vi "OP_Print_TPS_cluster0913.vi"() -> ()   [LabVIEW 2013]
uses:
  <vilib>/addons/database/Connection.llb/DB Tools Open Connec (Path).vi
  <vilib>/addons/database/Connection.llb/Conn Execute.vi
  <vilib>/addons/database/Recordset.llb/Rec Fetch Recordset Data (R).vi
  <vilib>/addons/database/Recordset.llb/Rec Destroy - Connection.vi
  <userlib>/caLab/Private/Get_PV-1D.vi
  <userlib>/caLab/Private/Get_PV.vi
  <vilib>/addons/database/NI_Database_API.lvlib
panel:
  in  "last ? Hrs":dbl=12.0 min=1.0 max=24.0 step=1.0
  out "error out 2":errorcluster
  out "x = y?":bool
  out "NOW time":string="21:22:35"
  out "NOW date":string="2017/09/13"
  in  "Save Button":bool
  out "error out 3":errorcluster
  in  "stop":bool
  out "time kickeron":string="21:11:02"
  out "date kickeron":string="2017/09/13"
  out "Cluster":T1={"SR Fill Pattern"=array[864 elements], "Beam Current(mA"=301.29559, "Beam Lifetime(min)"=467.3623843429031, "Beamsize X(um)"=61.81771808059018, "Beamsize Y(um)"=34.43346871436747, "Tune X(from BPM)"=0.0, "Tune Y(from BPM)"=0.0, "Mode"="Top-Up", "NuX(from BBF) "=0.15280663925802224, "NuY(from BBF)"=0.22496346361412184, "IU22-23gap(R)"=7.0, "IU22-05gap(R)"=7.28, "IU22-05M"=TRUE, "IU22A-09gap(R)"=8.058, "IU22A-09M"=TRUE, "IU22B-09gap(R)"=40.001, "IU22B-09M"=FALSE, "IUT22-21gap(R)"=7.0, "IUT22-21M"=TRUE, "IU22-23M"=TRUE, "IU22A-25gap(R)"=7.0, "IU22A-25M"=TRUE, "IU22B-25gap(R)"=40.0, "IU22B-25M"=FALSE, "EPU48A-41gap(R)"=65.0, "EPU48A-41gM"=FALSE, "EPU48B-41gap(R)"=44.99995, "EPU48B-41gM"=TRUE, "EPU46-45gap(R)"=65.00120000000001, "EPU46-45gM"=FALSE, "EPU48A-41phase(R)"=0.0009500000000000001, "EPU48B-41phase(R)"=0.0, "EPU46-45phase(R)"=0.0, "Grid volt.(V)(S)"=33.0, "Gun mode"="MBM", "Mod.3 HV(kV)(S)"=35.519999999999996, "SR"="SR_DMB_2017_0910_1700LOCO.data", "BR"="Booster_JT_2017_0714_1140.data", "Linac"="Linac_2017_0413_1015.data", "LTB"="LTB_JT_2017_0828_1050.data", "BTS"="BTS_2017_0911_0610.data", "RF2 remote"=TRUE, "RF2 OP mode"=TRUE, "RF2 phase.(S)"=-36.2, "RF Freq.(s)"=499655122.5507494, "RF2 gap volt.(S)"=1400.0, "RF3 remote"=TRUE, "RF3 OP mode"=TRUE, "RF3 phase.(S)"=9.000000000000004, "RF3 gap volt.(S)"=1400.0, "BBF V"=TRUE, "BBF H"=TRUE, "BR ext. kicker1(kV)"=17.666, "BR ext. kicker2(kV)"=17.666, "BR ext. sep.1(V)"=322.14, "BR ext. sep.2(V)"=441.1, "BR inj. sep.(V)"=104.95, "BR inj. kicker(kV)"=12.131749999999993, "SR kicker4(kV)"=8.133, "SR kicker3(kV)"=7.798, "SR kicker2(kV)"=8.259, "SR kicker1(kV)"=8.2, "SR inj. sep.2(V)"=397.2, "SR inj. sep.1(V)"=398.04, "Bucket Start"=100.0, "Bucket Last"=600.0, "Bucket Step"=10.0, "Orbit ILK(P)"=TRUE, "IU22-05 Hutch Enable"=TRUE, "IU22A-09M Hutch Enable"=TRUE, "IUT22-21M Hutch Enable"=TRUE, "IU22-23M Hutch Enable"=TRUE, "IU22A-25M Hutch Enable"=TRUE, "EPU48A-41M Hutch Enable"=FALSE, "EPU46-45M Hutch Enable"=FALSE, "EPU46-45 FE Enable"=TRUE, "EPU48A-41 FE Enable"=TRUE, "IU22A-25 FE Enable"=TRUE, "IU22-23 FE Enable"=TRUE, "IUT22-21 FE Enable"=TRUE, "IU22A-09 FE Enable"=TRUE, "IU22-05 FE Enable"=TRUE, "EPU48A-41pM"=FALSE, "EPU48B-41pM"=TRUE, "EPU46-45pM"=FALSE, "Gun volt.(V)(S)"=23.5, "Width count"=30.0, "2ns step"=0.0, "10ps delay"=150.0, "phase shifter"=130.0021, "Taper"=1.0899999999999999, "05XBPMX 1"=-12.071, "09XBPMX 1"=236.232, "21XBPMX 1"=109.949, "23XBPMX 1"=-54.123000000000005, "25XBPMX 1"=836.426, "41XBPMX 1"=-393.619, "45XBPMX 1"=-542.557, "05XBPMY 1"=49.623, "09XBPMY 1"=-49.685, "21XBPMY 1"=1810.249, "23XBPMY 1"=8.221, "25XBPMY 1"=-161.43800000000002, "41XBPMY 1"=188.45000000000002, "45XBPMY 1"=-785.827, "FOFB H"="On", "FOFB V"="On", "time string"="21:22:35", "date"="2017/09/13", "date (last kicker ON)"="2017/09/13", "time string (last kicker ON)"="21:11:02", "BPMX Graph"={[1, 2, 3, 4, 5, 6, 7, 8, 9, 10, 11, 12, 13, 14, 15, 16, 17, 18, 19, 20, 21, 22, 23, 24, 25, 26, 27, 28, 29, 30, 31, 32, 33, 34, 35, 36, 37, 38, 39, 40, 41, 42, 43, 44, 45, 46, 47, 48, 49, 50, 51, 52, 53, 54, 55, 56, 57, 58, 59, 60, 61, 62, 63, 64, 65, 66, 67, 68, 69, 70, 71, 72, 73, 74, 75, 76, 77, 78, 79, 80, 81, 82, 83, 84, 85, 86, 87, 88, 89, 90, 91, 92, 93, 94, 95, 96, 97, 98, 99, 100, 101, 102, 103, 104, 105, 106, 107, 108, 109, 110, 111, 112, 113, 114, 115, 116, 117, 118, 119, 120, 121, 122, 123, 124, 125, 126, 127, 128, 129, 130, 131, 132, 133, 134, 135, 136, 137, 138, 139, 140, 141, 142, 143, 144, 145, 146, 147, 148, 149, 150, 151, 152, 153, 154, 155, 156, 157, 158, 159, 160, 161, 162, 163, 164, 165, 166, 167, 168, 169, 170, 171, 172, 173, 174], "1rst Value (number)"=[-57.953, -16.830000000000002, -69.81400000000001, 33.217, 55.747, -102.116, 112.23700000000001, -53.109, -8.106, -108.797, 42.098, -26.618000000000002, 23.191, -14.290000000000001, -1.155, -135.518, -122.34, 81.94200000000001, -31.955000000000002, -107.23100000000001, 144.648, -41.501, -20.927, -71.483, 72.117, 174.239, 163.291, 218.172, -123.111, -19.648, 721.419, 453.44, -205.66400000000002, 29.594, 134.439, -81.831, 78.56700000000001, 81.661, 6.593, -174.97, 3.722, 159.74, -88.646, 74.924, 15.269, -34.265, -113.105, -24.846, 66.414, -131.589, 93.44500000000001, 99.491, -12.985, -180.05100000000002, 131.165, 37.079, -154.526, 160.38400000000001, 49.599000000000004, 24.96, -73.793, 85.367, 37.467, -10.198, 89.935, -39.093, 45.050000000000004, -60.443, 91.7, -89.60600000000001, -338.463, -13.786, -319.98900000000003, -247.719, -134.31, 117.925, -10.984, -69.336, 71.378, -119.991, 35.43, -76.868, 56.546, -1.875, -582.236, -130.956, -298.747, -39.141, 76.82900000000001, 82.033, -47.447, 68.075, 11.526, -161.376, 200.095, -3.3000000000000003, -170.391, -174.619, -59.896, 50.463, -167.593, 164.144, 6.708, -52.142, -152.178, 67.056, 8.861, -173.928, 197.31, 48.799, -71.952, -62.230000000000004, -4.128, 137.421, -127.104, 79.596, 56.283, -67.373, -122.31400000000001, 36.139, 42.783, -82.897, 55.373000000000005, 14.632, -53.128, -78.393, 32.919000000000004, -27.649, -194.787, 148.28300000000002, 205.038, -156.17600000000002, -87.652, -24.492, 101.044, -122.638, 98.552, 5.809, 62.325, -64.294, 38.297000000000004, 46.068, 274.628, 436.098, -130.642, -298.747, 133.037, 11.423, -153.334, 114.726, 76.023, -90.009, 92.394, 59.627, -74.368, -118.376, 43.591, 66.153, -129.306, 168.713, 4.539, -35.064, -130.217, 42.444, 59.192, -125.98400000000001, 147.53, 66.584, -28.801000000000002, -176.53, 75.164, 77.199, -57.284, -9.878]}, "BPMY Graph"={[1, 2, 3, 4, 5, 6, 7, 8, 9, 10, 11, 12, 13, 14, 15, 16, 17, 18, 19, 20, 21, 22, 23, 24, 25, 26, 27, 28, 29, 30, 31, 32, 33, 34, 35, 36, 37, 38, 39, 40, 41, 42, 43, 44, 45, 46, 47, 48, 49, 50, 51, 52, 53, 54, 55, 56, 57, 58, 59, 60, 61, 62, 63, 64, 65, 66, 67, 68, 69, 70, 71, 72, 73, 74, 75, 76, 77, 78, 79, 80, 81, 82, 83, 84, 85, 86, 87, 88, 89, 90, 91, 92, 93, 94, 95, 96, 97, 98, 99, 100, 101, 102, 103, 104, 105, 106, 107, 108, 109, 110, 111, 112, 113, 114, 115, 116, 117, 118, 119, 120, 121, 122, 123, 124, 125, 126, 127, 128, 129, 130, 131, 132, 133, 134, 135, 136, 137, 138, 139, 140, 141, 142, 143, 144, 145, 146, 147, 148, 149, 150, 151, 152, 153, 154, 155, 156, 157, 158, 159, 160, 161, 162, 163, 164, 165, 166, 167, 168, 169, 170, 171, 172, 173, 174], "1rst Value (number)"=[-151.316, -17.054000000000002, -19.178, 120.799, -59.688, 21.818, 7.809, -29.198, 24.311, 16.134, -40.005, -27.325, 53.925000000000004, 3.1670000000000003, -9.254, 61.293, -34.105000000000004, 94.741, -29.063, -23.54, 22.793, 14.087, -38.574, 36.56, -99.245, -0.044, 48.661, 33.093, -212.454, -68.398, 390.704, 121.525, -58.935, -19.379, 2.579, -18.495, 19.617, -37.129, 48.386, 12.363, -36.386, 3.988, 67.735, -11.383000000000001, 4.172, -13.203, 10.164, -0.589, -22.969, 30.752, -38.915, 41.105000000000004, -21.456, -4.901, 29.631, -9.992, -32.032000000000004, 12.132, -68.125, 97.674, -58.86, 66.602, -68.949, 58.512, -42.012, 22.742, -15.959, 12.297, 5.471, -82.755, 65.11, 15.540000000000001, -166.881, -18.198, 7.187, -10.503, 30.153000000000002, -70.941, -3.086, 7.163, -7.828, -18.855, 26.188, -7.574, 38.271, 0.135, -13.549, 40.546, 139.87800000000001, 4.58, -2.962, -6.871, 5.808, 0.435, 13.713000000000001, -7.65, -7.087, -2.88, 14.262, -32.895, 32.566, -5.7620000000000005, -44.698, 76.731, -22.138, 22.336000000000002, -6.075, -10.424, 12.001, -9.495000000000001, 18.714, -1.697, 7.412, -43.832, 47.095, -41.426, 2.965, 43.068, 29.560000000000002, -31.904, 28.699, -0.466, -7.138, -5.288, -15.559000000000001, 34.502, -45.603, -18.644000000000002, -3.043, -37.238, -6.869, -15.336, -4.0600000000000005, 13.134, -43.802, 53.087, -14.268, -32.236000000000004, 35.516, -16.788, 25.02, -56.714, 59.035000000000004, 117.801, 64.776, -29.192, -39.944, 137.099, -65.81700000000001, 24.237000000000002, -41.801, 16.21, 15.972, -22.743000000000002, 31.377, 18.596, 7.515000000000001, -19.796, 10.161, 1.0070000000000001, -7.114, -12.046, -4.223, 21.048000000000002, -8.239, -20.592, -8.097, 90.321, -136.733, 37.556, 84.604, -63.991, 30.307000000000002, 1.127]}, "Radio Buttons 2"=enum."absolute", "09XBPMX 2"="-47.22", "09XBPMY 2"="-3.76", "05XBPMY 2"="-491.14", "05XBPMX 2"="-472.70", "21XBPMY 2"=" closed", "21XBPMX 2"=" PAB ", "23XBPMY 2"="188.03", "23XBPMX 2"="-8.61", "25XBPMY 2"="5165.53", "25XBPMX 2"="2146.38", "41XBPMY 2"=" closed", "41XBPMX 2"=" Hutch ", "45XBPMX 2"=" Hutch ", "45XBPMY 2"=" closed", "05 mode"="Follow", "09A mode"="Follow", "09B mode"="Follow", "21 mode"="Follow", "23 mode"="Follow", "25A mode"="Follow", "25B mode"="Follow", "41A mode"="Follow", "41B mode"="Follow", "46 mode"="Follow", "BeamCurrent History"={"BPM NO.  1_172"=array[4320 elements], array[4320 elements]}, "SR Beam Current in            hours"=12.0} {"SR Beam Current in            hours" min=1.0 max=24.0 step=1.0 format="%#_2f"; "45XBPMY 1" format="%#.2f"; "41XBPMY 1" format="%#.2f"; "25XBPMY 1" format="%#.2f"; "23XBPMY 1" format="%#.2f"; "21XBPMY 1" format="%#.2f"; "09XBPMY 1" format="%#.2f"; "05XBPMY 1" format="%#.2f"; "45XBPMX 1" format="%#.2f"; "41XBPMX 1" format="%#.2f"; "25XBPMX 1" format="%#.2f"; "23XBPMX 1" format="%#.2f"; "21XBPMX 1" format="%#.2f"; "09XBPMX 1" format="%#.2f"; "05XBPMX 1" format="%#.2f"; "Taper" format="%#.4f"; "phase shifter" format="%#.3f"; "10ps delay" format="%#.1f"; "2ns step" format="%#.1f"; "Width count" format="%#.1f"; "Gun volt.(V)(S)" format="%#.1f"; "Bucket Step" format="%#.2f"; "Bucket Last" format="%#.2f"; "Bucket Start" format="%#.2f"; "BR ext. kicker1(kV)" format="%#.2f"; "BR ext. kicker2(kV)" format="%#.2f"; "BR ext. sep.1(V)" format="%#.2f"; "BR ext. sep.2(V)" format="%#.2f"; "BR inj. sep.(V)" format="%#.3f"; "BR inj. kicker(kV)" format="%#.3f"; "SR kicker4(kV)" format="%#.2f"; "SR kicker3(kV)" format="%#.2f"; "SR kicker2(kV)" format="%#.2f"; "SR kicker1(kV)" format="%#.2f"; "SR inj. sep.2(V)" format="%#.2f"; "SR inj. sep.1(V)" format="%#.2f"; "RF3 gap volt.(S)" format="%#.0f"; "RF3 phase.(S)" format="%#.1f"; "RF2 gap volt.(S)" format="%#.0f"; "RF Freq.(s)" format="%#.1f"; "RF2 phase.(S)" format="%#.1f"; "Mod.3 HV(kV)(S)" format="%#.3f"; "Grid volt.(V)(S)" format="%#.1f"; "EPU46-45phase(R)" format="%#.4f"; "EPU48B-41phase(R)" format="%#.4f"; "EPU48A-41phase(R)" format="%#.4f"; "EPU46-45gap(R)" format="%#.4f"; "EPU48B-41gap(R)" format="%#.4f"; "EPU48A-41gap(R)" format="%#.4f"; "IU22B-25gap(R)" format="%#.4f"; "IU22A-25gap(R)" format="%#.4f"; "IUT22-21gap(R)" format="%#.4f"; "IU22B-09gap(R)" format="%#.4f"; "IU22A-09gap(R)" format="%#.4f"; "IU22-05gap(R)" format="%#.4f"; "IU22-23gap(R)" format="%#.4f"; "NuY(from BBF)" format="%#.4f"; "NuX(from BBF)" format="%#.4f"; "Tune Y(from BPM)" format="%#.4f"; "Tune X(from BPM)" format="%#.4f"; "Beamsize Y(um)" format="%#.2f"; "Beamsize X(um)" format="%#.2f"; "Beam Lifetime(min)" format="%#.3f"; "Beam Current(mA" format="%#.3f"}
  out "date (last Gun ON)":string="2016/08/29"
  out "time string (last Gun ON)":string="23:28:50"
  out "Value Array (number) 7":dbl[](array[numeric])=[-12.071, 49.623, 236.232, -49.685, 109.949, 1810.249, -54.123000000000005, 8.221, 836.426, -161.43800000000002, -393.619, 188.45000000000002, -542.557, -785.827, -472.696, -491.142, -47.215, -3.761, 16.193, -29.476, -8.605, 188.026, 2146.382, 5165.525000000001, -28.331, 10.717, 132.828, -84.862]
  out "Value Array (number) 6":dbl[](array[numeric])=[7.28, 8.058, 40.001, 7.0, 7.0, 7.0, 40.0, 65.0, 0.0009500000000000001, 44.99995, 0.0, 65.00120000000001, 0.0, -1.0899999999999999, 130.0021]
  out "1rst Value (string) 2":string[](array[string])=["MBM", "33", "23.5", "350", "35.52", "22485", "22485", "62", "30", "0", "0", "200", "150"]
  out "Value Array (number) 5":dbl[](array[numeric])=[499654641.19275105, 1.0, 0.0, 1335.005102558433, 1400.0, -56.1, 1.0, 0.0, 1362.1066276040413, 1400.0, 160.0]
  out "1rst Value (string)":string[](array[string])=["Linac_2017_0413_1015.data", "LTB_JT_2017_0828_1050.data", "Booster_JT_2017_0714_1140.data", "BTS_2017_0911_0610.data", "SR_DMB_2017_0910_1700LOCO.data"]
  out "Value Array (number) 4":dbl[](array[numeric])=[499655122.5507494, 1.0, 0.0, 1326.2153542928932, 1400.0, -36.2, 1.0, 0.0, 1398.366426317367, 1400.0, 9.000000000000004]
  out "Value Array (number) 3":dbl[](array[numeric])=[0.0, 33.0, 23.5, 350.0, 35.519999999999996, 22485.0, 22485.0, 62.0, 30.0, 0.0, 0.0, 200.0, 150.0]
  out "Value Array (number) 2":dbl[](array[numeric])=[104.95, 12.131749999999993, 17.666, 17.666, 322.14, 441.1, 398.04, 397.2, 8.2, 8.259, 7.798, 8.133]
  out "Value Array (number)":dbl[](array[numeric])=[1.0, 301.29559, 467.3623843429031, 51.42904998385207, 28.64681257434898, 0.1761252446183953, 0.12524461839530332, 88.36853790283203, 130.0970458984375, 100.0, 600.0, 10.0]
  out "Orbit ILK(A)":bool
  out "Orbit INT. Ang Active":bool
  out "Orbit INT.Ang. On":bool
  out "Orbit INT. Pos Active":bool
  out "Orbit INT.Pos. On":bool
  out "SBM volt.(S)":dbl=350.0 format="%#.1f"
  out "MBM volt.(S)":dbl=23.5 format="%#.1f"
  in  "Copy Button":bool
  in  "Print Button":bool
  in  "Help Button":bool
  in  "Refresh Button":bool
  in  "Open Button":bool
  out "Gun WCM":dbl[](graph)
  out "BR Fill Pattern":dbl[](graph)
  # "TPS OP Handover Information"
  # "Others"
  # "Time："
  # "Valve  Status"
  # "follow"
  # "SM Status"
  # "歷史電流圖\ntrip次數?\n輻射劑量?\n平均氣壓\n目前最高累計劑量\n最近一次觸發時BR電流及WCM數值"
  # "TPS Operational Handover Information v1.3"
  # "SR Status"
  # "Feedback"
  # "Pulse Mag"
  # "LINAC"
  # "x8(ns)"
  # "x2(ns)"
  # "x0.01(ns)"
  # "RF Status"
  # "Hz"
  # "(kV)"
  # "(kV)"
  # "Changeliang@LOP.NSRRC"
  # "SR Fill Pattern"
  # "Lattice Files in using"
  # "ID &Beamline (R)"
  # "mode"
  # "Gap\nmm"
  # "Motor"
  # "Phase"
  # "FE/Hutch"
  # "phase\nshifter"
  # "Taper\n(enc)"
  # "XBPM1X\num"
  # "XBPM1Y\num"
  # "XBPM2X\num"
  # "XBPM2Y\num"
  # "05"
  # "09"
  # "21"
  # "23"
  # "25"
  # "41"
  # "45"
  # "SR Orbit"
  # "BPMX"
  # "BPMY"
  # "SR Beam Current History"
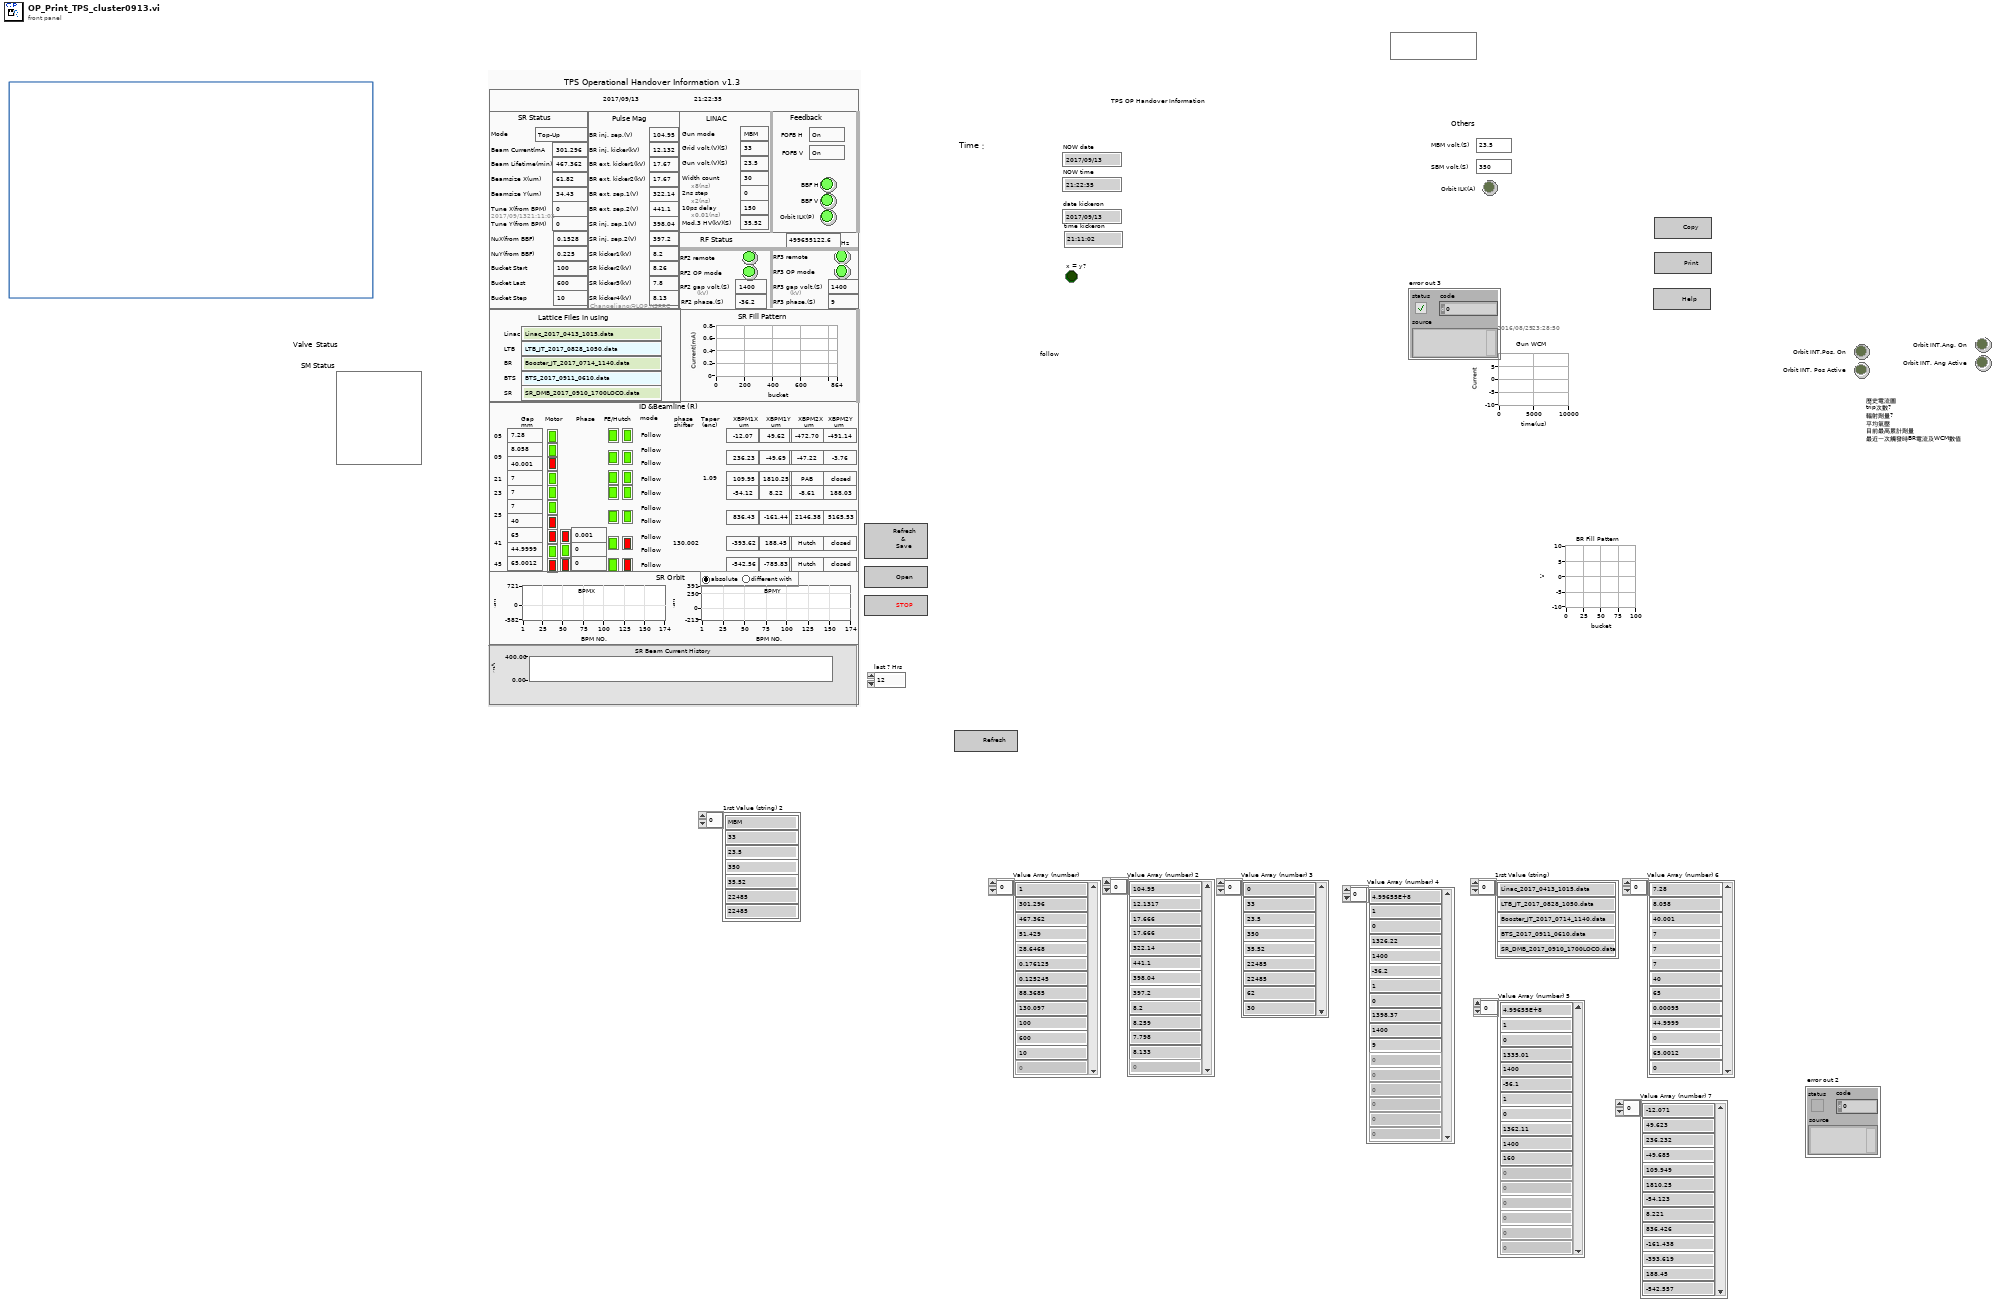
[diagram p1: front panel]
types:
  T1 = cluster{"SR Fill Pattern":dbl[], "Beam Current(mA":dbl, "Beam Lifetime(min)":dbl, "Beamsize X(um)":dbl, "Beamsize Y(um)":dbl, "Tune X(from BPM)":dbl, "Tune Y(from BPM)":dbl, "Mode":string, "NuX(from BBF) ":dbl, "NuY(from BBF)":dbl, "IU22-23gap(R)":dbl, "IU22-05gap(R)":dbl, "IU22-05M":bool, "IU22A-09gap(R)":dbl, "IU22A-09M":bool, "IU22B-09gap(R)":dbl, "IU22B-09M":bool, "IUT22-21gap(R)":dbl, "IUT22-21M":bool, "IU22-23M":bool, "IU22A-25gap(R)":dbl, "IU22A-25M":bool, "IU22B-25gap(R)":dbl, "IU22B-25M":bool, "EPU48A-41gap(R)":dbl, "EPU48A-41gM":bool, "EPU48B-41gap(R)":dbl, "EPU48B-41gM":bool, "EPU46-45gap(R)":dbl, "EPU46-45gM":bool, "EPU48A-41phase(R)":dbl, "EPU48B-41phase(R)":dbl, "EPU46-45phase(R)":dbl, "Grid volt.(V)(S)":dbl, "Gun mode":string, "Mod.3 HV(kV)(S)":dbl, "SR":string, "BR":string, "Linac":string, "LTB":string, "BTS":string, "RF2 remote":bool, "RF2 OP mode":bool, "RF2 phase.(S)":dbl, "RF Freq.(s)":dbl, "RF2 gap volt.(S)":dbl, "RF3 remote":bool, "RF3 OP mode":bool, "RF3 phase.(S)":dbl, "RF3 gap volt.(S)":dbl, "BBF V":bool, "BBF H":bool, "BR ext. kicker1(kV)":dbl, "BR ext. kicker2(kV)":dbl, "BR ext. sep.1(V)":dbl, "BR ext. sep.2(V)":dbl, "BR inj. sep.(V)":dbl, "BR inj. kicker(kV)":dbl, "SR kicker4(kV)":dbl, "SR kicker3(kV)":dbl, "SR kicker2(kV)":dbl, "SR kicker1(kV)":dbl, "SR inj. sep.2(V)":dbl, "SR inj. sep.1(V)":dbl, "Bucket Start":dbl, "Bucket Last":dbl, "Bucket Step":dbl, "Orbit ILK(P)":bool, "IU22-05 Hutch Enable":bool, "IU22A-09M Hutch Enable":bool, "IUT22-21M Hutch Enable":bool, "IU22-23M Hutch Enable":bool, "IU22A-25M Hutch Enable":bool, "EPU48A-41M Hutch Enable":bool, "EPU46-45M Hutch Enable":bool, "EPU46-45 FE Enable":bool, "EPU48A-41 FE Enable":bool, "IU22A-25 FE Enable":bool, "IU22-23 FE Enable":bool, "IUT22-21 FE Enable":bool, "IU22A-09 FE Enable":bool, "IU22-05 FE Enable":bool, "EPU48A-41pM":bool, "EPU48B-41pM":bool, "EPU46-45pM":bool, "Gun volt.(V)(S)":dbl, "Width count":dbl, "2ns step":dbl, "10ps delay":dbl, "phase shifter":dbl, "Taper":dbl, "05XBPMX 1":dbl, "09XBPMX 1":dbl, "21XBPMX 1":dbl, "23XBPMX 1":dbl, "25XBPMX 1":dbl, "41XBPMX 1":dbl, "45XBPMX 1":dbl, "05XBPMY 1":dbl, "09XBPMY 1":dbl, "21XBPMY 1":dbl, "23XBPMY 1":dbl, "25XBPMY 1":dbl, "41XBPMY 1":dbl, "45XBPMY 1":dbl, "FOFB H":string, "FOFB V":string, "time string":string, "date":string, "date (last kicker ON)":string, "time string (last kicker ON)":string, "BPMX Graph":cluster{i32[], "1rst Value (number)":dbl[]}, "BPMY Graph":cluster{i32[], "1rst Value (number)":dbl[]}, "Radio Buttons 2":enum32{"absolute", "different with"}, "09XBPMX 2":string, "09XBPMY 2":string, "05XBPMY 2":string, "05XBPMX 2":string, "21XBPMY 2":string, "21XBPMX 2":string, "23XBPMY 2":string, "23XBPMX 2":string, "25XBPMY 2":string, "25XBPMX 2":string, "41XBPMY 2":string, "41XBPMX 2":string, "45XBPMX 2":string, "45XBPMY 2":string, "05 mode":string, "09A mode":string, "09B mode":string, "21 mode":string, "23 mode":string, "25A mode":string, "25B mode":string, "41A mode":string, "41B mode":string, "46 mode":string, "BeamCurrent History":cluster{"BPM NO.  1_172":dbl[], dbl[]}, "SR Beam Current in            hours":dbl}
  T2 = typedef "NI_Database_API.lvlib/Conn ObjectReference.ctl" = refnum<k1>
  T3 = typedef "NI_Database_API.lvlib/Rec ObjectReference.ctl" = refnum<k1>
  T4 = cluster{"SR Fill Pattern":dbl[], "Beam Current(mA":dbl, "Beam Lifetime(min)":dbl, "Beamsize X(um)":dbl, "Beamsize Y(um)":dbl, "Tune X(from BPM)":dbl, "Tune Y(from BPM)":dbl, "Mode":string, "NuX(from BBF) ":dbl, "NuY(from BBF)":dbl, "IU22-23gap(R)":dbl, "IU22-05gap(R)":dbl, "IU22-05M":bool, "IU22A-09gap(R)":dbl, "IU22A-09M":bool, "IU22B-09gap(R)":dbl, "IU22B-09M":bool, "IUT22-21gap(R)":dbl, "IUT22-21M":bool, "IU22-23M":bool, "IU22A-25gap(R)":dbl, "IU22A-25M":bool, "IU22B-25gap(R)":dbl, "IU22B-25M":bool, "EPU48A-41gap(R)":dbl, "EPU48A-41gM":bool, "EPU48B-41gap(R)":dbl, "EPU48B-41gM":bool, "EPU46-45gap(R)":dbl, "EPU46-45gM":bool, "EPU48A-41phase(R)":dbl, "EPU48B-41phase(R)":dbl, "EPU46-45phase(R)":dbl, "Grid volt.(V)(S)":dbl, "Gun mode":string, "Mod.3 HV(kV)(S)":dbl, "SR":string, "BR":string, "Linac":string, "LTB":string, "BTS":string, "RF2 remote":bool, "RF2 OP mode":bool, "RF2 phase.(S)":dbl, "RF Freq.(s)":dbl, "RF2 gap volt.(S)":dbl, "RF3 remote":bool, "RF3 OP mode":bool, "RF3 phase.(S)":dbl, "RF3 gap volt.(S)":dbl, "BBF V":bool, "BBF H":bool, "BR ext. kicker1(kV)":dbl, "BR ext. kicker2(kV)":dbl, "BR ext. sep.1(V)":dbl, "BR ext. sep.2(V)":dbl, "BR inj. sep.(V)":dbl, "BR inj. kicker(kV)":dbl, "SR kicker4(kV)":dbl, "SR kicker3(kV)":dbl, "SR kicker2(kV)":dbl, "SR kicker1(kV)":dbl, "SR inj. sep.2(V)":dbl, "SR inj. sep.1(V)":dbl, "Bucket Start":dbl, "Bucket Last":dbl, "Bucket Step":dbl, "Orbit ILK(P)":bool, "IU22-05 Hutch Enable":bool, "IU22A-09M Hutch Enable":bool, "IUT22-21M Hutch Enable":bool, "IU22-23M Hutch Enable":bool, "IU22A-25M Hutch Enable":bool, "EPU48A-41M Hutch Enable":bool, "EPU46-45M Hutch Enable":bool, "EPU46-45 FE Enable":bool, "EPU48A-41 FE Enable":bool, "IU22A-25 FE Enable":bool, "IU22-23 FE Enable":bool, "IUT22-21 FE Enable":bool, "IU22A-09 FE Enable":bool, "IU22-05 FE Enable":bool, "EPU48A-41pM":bool, "EPU48B-41pM":bool, "EPU46-45pM":bool, "Gun volt.(V)(S)":dbl, "Width count":dbl, "2ns step":dbl, "10ps delay":dbl, "phase shifter":dbl, "Taper":dbl, "05XBPMX 1":dbl, "09XBPMX 1":dbl, "21XBPMX 1":dbl, "23XBPMX 1":dbl, "25XBPMX 1":dbl, "41XBPMX 1":dbl, "45XBPMX 1":dbl, "05XBPMY 1":dbl, "09XBPMY 1":dbl, "21XBPMY 1":dbl, "23XBPMY 1":dbl, "25XBPMY 1":dbl, "41XBPMY 1":dbl, "45XBPMY 1":dbl, "FOFB H":string, "FOFB V":string, "time string":string, "date":string, "date (last kicker ON)":string, "time string (last kicker ON)":string, "BPMX Graph":cluster{i32[], "1rst Value (number)":dbl[]}, "BPMY Graph":cluster{i32[], "1rst Value (number)":dbl[]}, "Radio Buttons 2":enum32{"absolute", "different with"}, "09XBPMX 2":string, "09XBPMY 2":string, "05XBPMY 2":string, "05XBPMX 2":string, "21XBPMY 2":string, "21XBPMX 2":string, "23XBPMY 2":string, "23XBPMX 2":string, "25XBPMY 2":string, "25XBPMX 2":string, "41XBPMY 2":string, "41XBPMX 2":string, "45XBPMX 2":string, "45XBPMY 2":string, "05 mode":string, "09A mode":string, "09B mode":string, "21 mode":string, "23 mode":string, "25A mode":string, "25B mode":string, "41A mode":string, "41B mode":string, "46 mode":string, "BeamCurrent History":cluster{"BPM NO.  1_172":dbl[], dbl[]}, "SR Beam Current in Last           Hrs":dbl}
  T5 = typedef "imagedata.ctl" = cluster{"image type":i32, "image depth":i32, "image":u8[], "mask":u8[], "colors":u32[], "Rectangle":cluster{"left":i16, "top":i16, "right":i16, "bottom":i16}}
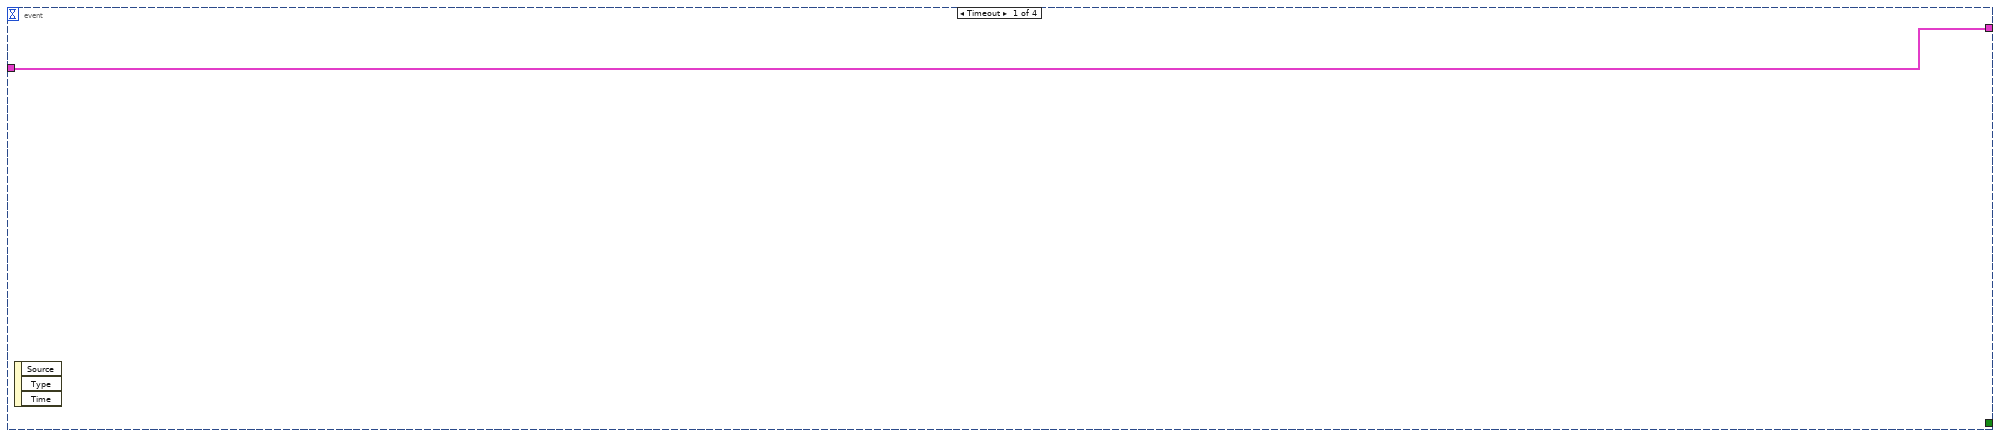
[diagram p4: hidden frame]
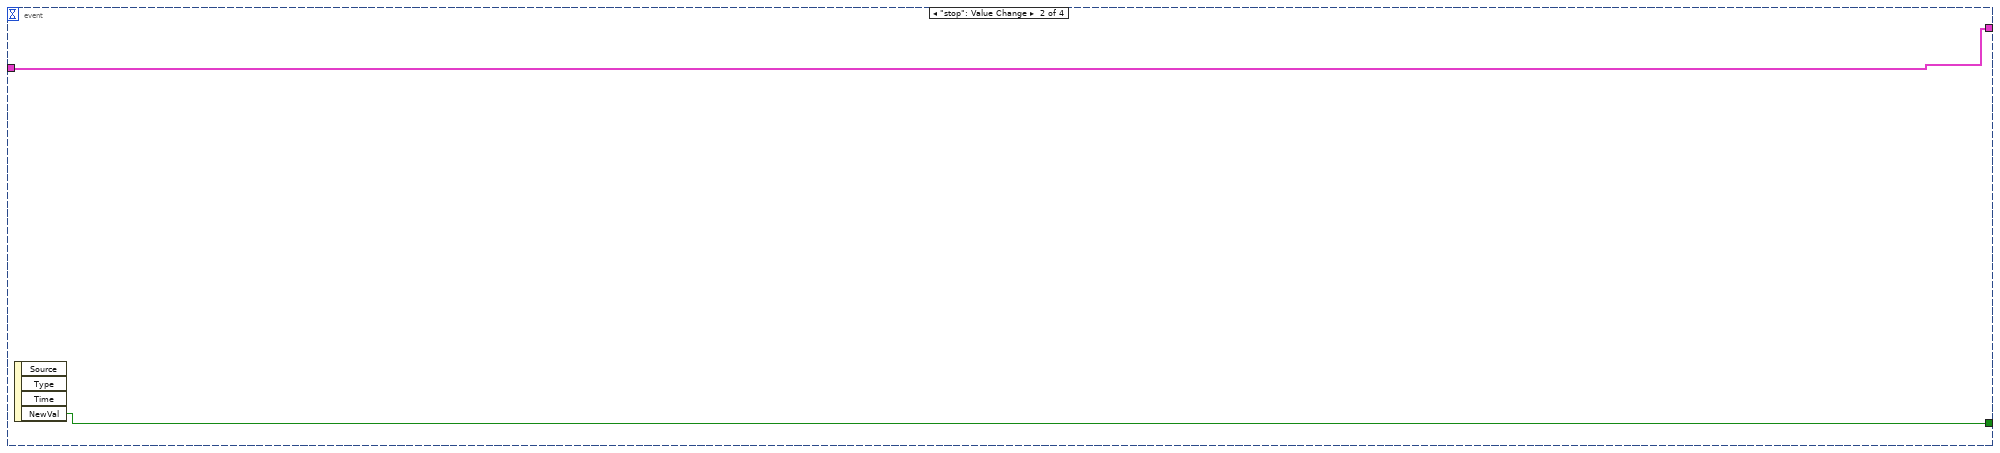
[diagram p5: hidden frame]
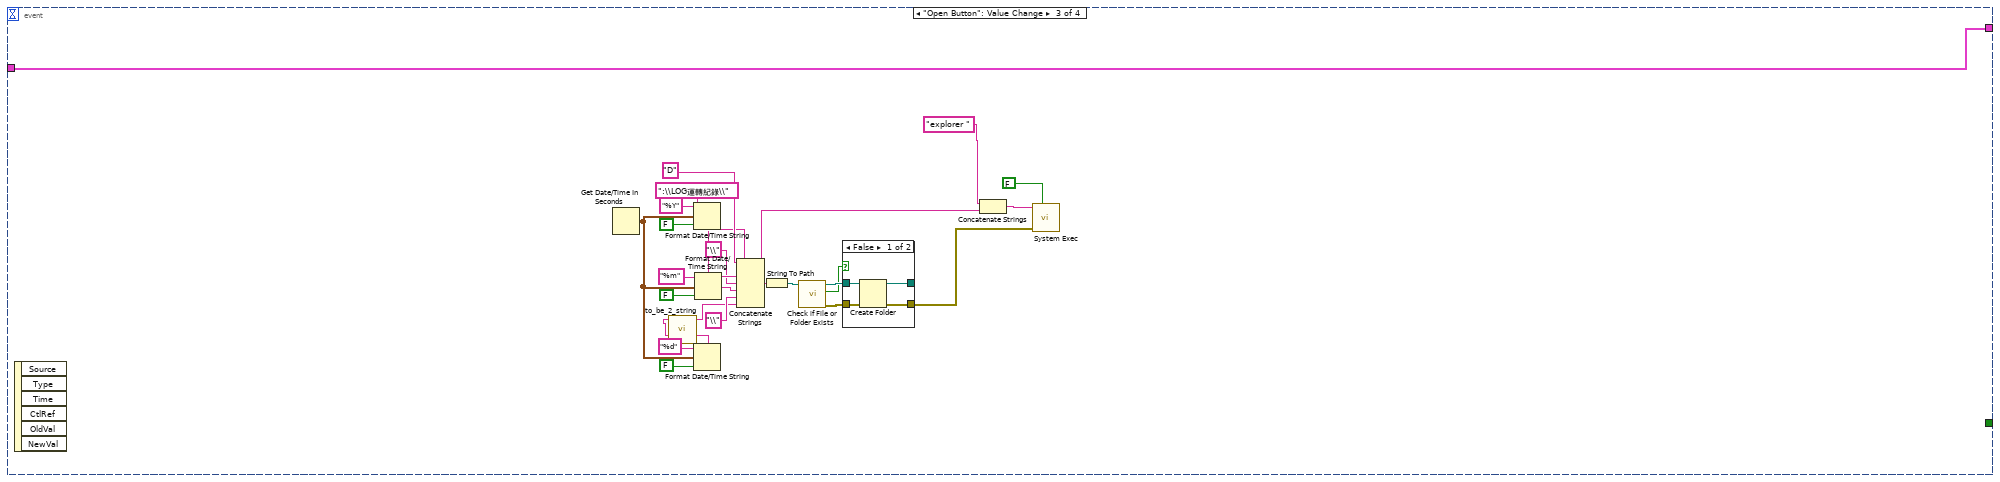
[diagram p6: hidden frame]
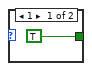
[diagram p9: hidden frame]
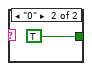
[diagram p12: hidden frame]
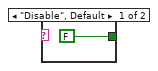
[diagram p13: hidden frame]
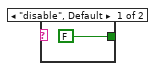
[diagram p14: hidden frame]
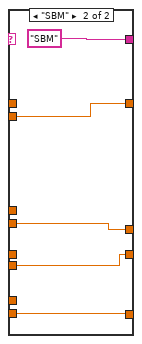
[diagram p15: hidden frame]
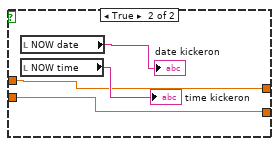
[diagram p16: hidden frame]
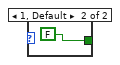
[diagram p17: hidden frame]
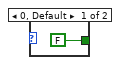
[diagram p18: hidden frame]
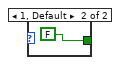
[diagram p19: hidden frame]
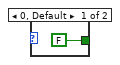
[diagram p20: hidden frame]
diagram:
  (unwired) string[] ["FE-DI-XBPM-051:SA:SA_X_MONITOR", "FE-DI-XBPM-051:SA:SA_Y_MONITOR", "FE-DI-XBPM-091:SA:SA_X_MONITOR", "FE-DI-XBPM-091:SA:SA_Y_MONITOR", "FE-DI-XBPM-211:SA:SA_X_MONITOR", "FE-DI-XBPM-211:SA:SA_Y_MONITOR", "FE-DI-XBPM-231:SA:SA_X_MONITOR", "FE-DI-XBPM-231:SA:SA_Y_MONITOR", "FE-DI-XBPM-251:SA:SA_X_MONITOR", "FE-DI-XBPM-251:SA:SA_Y_MONITOR", "FE-DI-XBPM-411:SA:SA_X_MONITOR", "FE-DI-XBPM-411:SA:SA_Y_MONITOR", "FE-DI-XBPM-451:SA:SA_X_MONITOR", "FE-DI-XBPM-451:SA:SA_Y_MONITOR"]
  (unwired) string[] ["LI-VA-VAL-01:STA:POS", "LI-VA-VAL-02:STA:POS", "LI-VA-VAL-03:STA:POS", "LI-VA-VAL-04:STA:POS", "LI-VA-VAL-05:STA:POS"]
  (unwired) string[] ["SR-DI-SOFB-H:getStatus", "SR-DI-SOFB-V:getStatus", "IGPF:TPSX:FBCTRL", "IGPF:TPSY:FBCTRL", "SR-DI-FOFB-H:getStatus", "SR-DI-FOFB-V:getStatus"]
  # "FE-DI-XBPM-051:SA:SA_Y_MONITOR"
  # "FE-DI-XBPM-051:SA:SA_X_MONITOR"
  # "TPS-SR-052:bpm4:ilk:enabled"
  # "0 為OPEN"
  # "VALVE(EPICS)"
  n1 = local read "last ? Hrs"() -> (w1:dbl)
  n2 = Multiply(x=3600.0 ("y"), y=w1) -> (x*y=w26:dbl)
  n3 = Get Date/Time In Seconds() -> (seconds since 1Jan1904=w36:timestamp)
  n4 = Subtract(x=w36, y=w26) -> (x-y=w35:timestamp)
  n5 = call "TimeToString.vi"("Time Stamp Control"=w36) -> ("result string"=w28:string)
  n6 = call "TimeToString.vi"("Time Stamp Control"=w35) -> ("result string"=w27:string)
  n7 = call <vilib>:"Application Directory.vi"() -> ("Application Directory"=w29:path)
  n8 = Build Path(base path=w29, name or relative path="DSN\\172-18-0-32.dsn") -> (appended path=w31:path)
  n9 = call-poly <vilib>:"DB Tools Open Connection.vi"("connection information"=w31) -> ("error out"=w19:errorcluster, "connection reference"=w18:T2)  [unwired: 7 in]
  n10 = Concatenate Strings("SELECT  float_val , smpl_time\nFROM sample \nwhere  channel_id = 104 and smpl_time between '" ("result string"), w27, "' ::timestamp and '" ("result string"), w28, "' ::timestamp" ("result string")) -> (w3:string)
  n11 = call-poly <vilib>:"DB Tools Execute Query.vi"("error in (no error)"=w19, "SQL query"=w3, "connection reference"=w18) -> ("error out"=w16:errorcluster, "recordset reference"=w17:T3)  [unwired: 5 in]
  n12 = control-ref of="BeamCurrent History"() -> (w32:refnum<vi>)
  n13 = To Double Precision Float(number=w36) -> (double precision float=w33:dbl)
  n14 = To Double Precision Float(number=w35) -> (double precision float=w34:dbl)
  n15 = call-poly <vilib>:"DB Tools Fetch Recordset Data.vi"("error in (no error)"=w16, "recordset reference"=w17) -> ("error out"=w14:errorcluster, "recordset data"=w11:variant[][], "recordset reference out"=w15:T3)  [unwired: 3 in]
  n16 = property on="Property Node" class="XYGraph (strict)"(reference=w32, "XScale.Maximum"=w33, "XScale.Minimum"=w34) -> ()  [unwired: 1 in, 2 out]
  n17 = call-poly <vilib>:"DB Tools Free Object.vi"("error in (no error)"=w14, "recordset reference"=w15) -> ("error out"=w12:errorcluster, "connection reference"=w13:T2)  [unwired: 8 in]
  n18 = Variant To Data(type=string[][] [], Variant=w11) -> (data=w9:string[][])  [unwired: 1 in, 1 out]
  n19 = call <vilib>:"DB Tools Close Connection.vi"("error in (no error)"=w12, "connection reference"=w13) -> ()  [unwired: 5 in, 1 out]
  n20 = Transpose 2D Array(2D array=w9) -> (transposed array=w7:string[][])
  n21 = Index Array(array=w7, index (row) #1=0 ("index (row)"), index (row) #2=1 ("index (row)")) -> (element #1=w21:string[], element #2=w24:string[])  [unwired: 2 in]
  n22 = Fract/Exp String To Number(string=w21) -> (number=w23:dbl[])  [unwired: 3 in, 1 out]
  n23 = for {
    tunnel: w24 -> [w40] mode=indexing
    tunnel: [w39] -> w22 mode=indexing
    n24 = Scan From String "Scan From String"(format string="%<%Y/%m/%d %p %I:%M:%S>T", input string=w40, initial scan location=u32 0, default 1=timestamp(-73814400 s since 1904-01-01)) -> (output 1=w43:timestamp)  [unwired: 1 in, 3 out]
    n25 = To Double Precision Float(number=w43) -> (double precision float=w39:dbl)
  }
  n26 = Bundle(w22, w23) -> (w2:cluster{dbl[], dbl[]})  [unwired: 1 in]
  n27 = while {
    shift-right: [w185] -> _
    shift-left: _ -> [w183]
    shift-right: [w184] -> _
    shift-left: _ -> [w182]
    shift-right: [w45] -> _
    shift-left: w2 -> [w44]
    stop <- "stop" stop-if-true
    w72 = string[] ["SR-ID-IU22-05:setECMode", "SR-ID-IU22A-09:setECMode", "SR-ID-IU22B-09:setECMode", "SR-ID-IUT22-21:setECMode", "SR-ID-IU22-23:setECMode", "SR-ID-IU22A-25:setECMode", "SR-ID-IU22B-25:setECMode", "SR-ID-EPU48A-41:setECMode", "SR-ID-EPU48B-41:setECMode", "SR-ID-EPU46-45:setECMode"]  # ID_mode
    w158 = string[] ["FE-05-PAB:Open", "FE-05-MGV:Open", "FE-05-FCV:Open", "FE-09-PAB:Open", "FE-09-MGV:Open", "FE-09-FCV:Open", "FE-21-PAB:Open", "FE-21-MGV:Open", "FE-21-FCV:Open", "FE-23-PAB:Open", "FE-23-PAB:Open", "FE-23-FCV:Open", "FE-25-PAB:Open", "FE-25-MGV:Open", "FE-25-FCV:Open", "FE-41-PAB:Open", "FE-41-MGV:Open", "FE-41-FCV:Open", "FE-45-PAB:Open", "FE-45-MGV:Open", "FE-45-FCV:Open"]  # PAB_MGV_FCV enable
    (unwired) "LI-DI-WCM:getWfCh1"
    (unwired) "SR-DI-FP:CurrentBuffer"
    w305 = i32[] [1, 2, 3, 4, 5, 6, 7, 8, 9, 10, 11, 12, 13, 14, 15, 16, 17, 18, 19, 20, 21, 22, 23, 24, 25, 26, 27, 28, 29, 30, 31, 32, 33, 34, 35, 36, 37, 38, 39, 40, 41, 42, 43, 44, 45, 46, 47, 48, 49, 50, 51, 52, 53, 54, 55, 56, 57, 58, 59, 60, 61, 62, 63, 64, 65, 66, 67, 68, 69, 70, 71, 72, 73, 74, 75, 76, 77, 78, 79, 80, 81, 82, 83, 84, 85, 86, 87, 88, 89, 90, 91, 92, 93, 94, 95, 96, 97, 98, 99, 100, 101, 102, 103, 104, 105, 106, 107, 108, 109, 110, 111, 112, 113, 114, 115, 116, 117, 118, 119, 120, 121, 122, 123, 124, 125, 126, 127, 128, 129, 130, 131, 132, 133, 134, 135, 136, 137, 138, 139, 140, 141, 142, 143, 144, 145, 146, 147, 148, 149, 150, 151, 152, 153, 154, 155, 156, 157, 158, 159, 160, 161, 162, 163, 164, 165, 166, 167, 168, 169, 170, 171, 172, 173, 174] ("Array 4")
    w303 = 0.001
    w301 = string[] ["SR-DI-BPM-011:Y", "SR-DI-BPM-012:Y", "SR-DI-BPM-013:Y", "SR-DI-BPM-014:Y", "SR-DI-BPM-015:Y", "SR-DI-BPM-016:Y", "SR-DI-BPM-017:Y", "SR-DI-BPM-021:Y", "SR-DI-BPM-022:Y", "SR-DI-BPM-023:Y", "SR-DI-BPM-024:Y", "SR-DI-BPM-025:Y", "SR-DI-BPM-026:Y", "SR-DI-BPM-027:Y", "SR-DI-BPM-031:Y", "SR-DI-BPM-032:Y", "SR-DI-BPM-033:Y", "SR-DI-BPM-034:Y", "SR-DI-BPM-035:Y", "SR-DI-BPM-036:Y", "SR-DI-BPM-037:Y", "SR-DI-BPM-041:Y", "SR-DI-BPM-042:Y", "SR-DI-BPM-043:Y", "SR-DI-BPM-044:Y", "SR-DI-BPM-045:Y", "SR-DI-BPM-046:Y", "SR-DI-BPM-047:Y", "SR-DI-BPM-048:Y", "SR-DI-BPM-050:Y", "SR-DI-BPM-051:Y", "SR-DI-BPM-052:Y", "SR-DI-BPM-053:Y", "SR-DI-BPM-054:Y", "SR-DI-BPM-055:Y", "SR-DI-BPM-056:Y", "SR-DI-BPM-057:Y", "SR-DI-BPM-061:Y", "SR-DI-BPM-062:Y", "SR-DI-BPM-063:Y", "SR-DI-BPM-064:Y", "SR-DI-BPM-065:Y", "SR-DI-BPM-066:Y", "SR-DI-BPM-067:Y", "SR-DI-BPM-071:Y", "SR-DI-BPM-072:Y", "SR-DI-BPM-073:Y", "SR-DI-BPM-074:Y", "SR-DI-BPM-075:Y", "SR-DI-BPM-076:Y", "SR-DI-BPM-077:Y", "SR-DI-BPM-081:Y", "SR-DI-BPM-082:Y", "SR-DI-BPM-083:Y", "SR-DI-BPM-084:Y", "SR-DI-BPM-085:Y", "SR-DI-BPM-086:Y", "SR-DI-BPM-087:Y", "SR-DI-BPM-091:Y", "SR-DI-BPM-092:Y", "SR-DI-BPM-093:Y", "SR-DI-BPM-094:Y", "SR-DI-BPM-095:Y", "SR-DI-BPM-096:Y", "SR-DI-BPM-097:Y", "SR-DI-BPM-101:Y", "SR-DI-BPM-102:Y", "SR-DI-BPM-103:Y", "SR-DI-BPM-104:Y", "SR-DI-BPM-105:Y", "SR-DI-BPM-106:Y", "SR-DI-BPM-107:Y", "SR-DI-BPM-111:Y", "SR-DI-BPM-112:Y", "SR-DI-BPM-113:Y", "SR-DI-BPM-114:Y", "SR-DI-BPM-115:Y", "SR-DI-BPM-116:Y", "SR-DI-BPM-117:Y", "SR-DI-BPM-121:Y", "SR-DI-BPM-122:Y", "SR-DI-BPM-123:Y", "SR-DI-BPM-124:Y", "SR-DI-BPM-125:Y", "SR-DI-BPM-126:Y", "SR-DI-BPM-127:Y", "SR-DI-BPM-128:Y", "SR-DI-BPM-130:Y", "SR-DI-BPM-131:Y", "SR-DI-BPM-132:Y", "SR-DI-BPM-133:Y", "SR-DI-BPM-134:Y", "SR-DI-BPM-135:Y", "SR-DI-BPM-136:Y", "SR-DI-BPM-137:Y", "SR-DI-BPM-141:Y", "SR-DI-BPM-142:Y", "SR-DI-BPM-143:Y", "SR-DI-BPM-144:Y", "SR-DI-BPM-145:Y", "SR-DI-BPM-146:Y", "SR-DI-BPM-147:Y", "SR-DI-BPM-151:Y", "SR-DI-BPM-152:Y", "SR-DI-BPM-153:Y", "SR-DI-BPM-154:Y", "SR-DI-BPM-155:Y", "SR-DI-BPM-156:Y", "SR-DI-BPM-157:Y", "SR-DI-BPM-161:Y", "SR-DI-BPM-162:Y", "SR-DI-BPM-163:Y", "SR-DI-BPM-164:Y", "SR-DI-BPM-165:Y", "SR-DI-BPM-166:Y", "SR-DI-BPM-167:Y", "SR-DI-BPM-171:Y", "SR-DI-BPM-172:Y", "SR-DI-BPM-173:Y", "SR-DI-BPM-174:Y", "SR-DI-BPM-175:Y", "SR-DI-BPM-176:Y", "SR-DI-BPM-177:Y", "SR-DI-BPM-181:Y", "SR-DI-BPM-182:Y", "SR-DI-BPM-183:Y", "SR-DI-BPM-184:Y", "SR-DI-BPM-185:Y", "SR-DI-BPM-186:Y", "SR-DI-BPM-187:Y", "SR-DI-BPM-191:Y", "SR-DI-BPM-192:Y", "SR-DI-BPM-193:Y", "SR-DI-BPM-194:Y", "SR-DI-BPM-195:Y", "SR-DI-BPM-196:Y", "SR-DI-BPM-197:Y", "SR-DI-BPM-201:Y", "SR-DI-BPM-202:Y", "SR-DI-BPM-203:Y", "SR-DI-BPM-204:Y", "SR-DI-BPM-205:Y", "SR-DI-BPM-206:Y", "SR-DI-BPM-207:Y", "SR-DI-BPM-208:Y", "SR-DI-BPM-210:Y", "SR-DI-BPM-211:Y", "SR-DI-BPM-212:Y", "SR-DI-BPM-213:Y", "SR-DI-BPM-214:Y", "SR-DI-BPM-215:Y", "SR-DI-BPM-216:Y", "SR-DI-BPM-217:Y", "SR-DI-BPM-221:Y", "SR-DI-BPM-222:Y", "SR-DI-BPM-223:Y", "SR-DI-BPM-224:Y", "SR-DI-BPM-225:Y", "SR-DI-BPM-226:Y", "SR-DI-BPM-227:Y", "SR-DI-BPM-231:Y", "SR-DI-BPM-232:Y", "SR-DI-BPM-233:Y", "SR-DI-BPM-234:Y", "SR-DI-BPM-235:Y", "SR-DI-BPM-236:Y", "SR-DI-BPM-237:Y", "SR-DI-BPM-241:Y", "SR-DI-BPM-242:Y", "SR-DI-BPM-243:Y", "SR-DI-BPM-244:Y", "SR-DI-BPM-245:Y", "SR-DI-BPM-246:Y", "SR-DI-BPM-247:Y"]  # sorted BPMY_174
    w300 = string[] ["SR-DI-BPM-011:X", "SR-DI-BPM-012:X", "SR-DI-BPM-013:X", "SR-DI-BPM-014:X", "SR-DI-BPM-015:X", "SR-DI-BPM-016:X", "SR-DI-BPM-017:X", "SR-DI-BPM-021:X", "SR-DI-BPM-022:X", "SR-DI-BPM-023:X", "SR-DI-BPM-024:X", "SR-DI-BPM-025:X", "SR-DI-BPM-026:X", "SR-DI-BPM-027:X", "SR-DI-BPM-031:X", "SR-DI-BPM-032:X", "SR-DI-BPM-033:X", "SR-DI-BPM-034:X", "SR-DI-BPM-035:X", "SR-DI-BPM-036:X", "SR-DI-BPM-037:X", "SR-DI-BPM-041:X", "SR-DI-BPM-042:X", "SR-DI-BPM-043:X", "SR-DI-BPM-044:X", "SR-DI-BPM-045:X", "SR-DI-BPM-046:X", "SR-DI-BPM-047:X", "SR-DI-BPM-048:X", "SR-DI-BPM-050:X", "SR-DI-BPM-051:X", "SR-DI-BPM-052:X", "SR-DI-BPM-053:X", "SR-DI-BPM-054:X", "SR-DI-BPM-055:X", "SR-DI-BPM-056:X", "SR-DI-BPM-057:X", "SR-DI-BPM-061:X", "SR-DI-BPM-062:X", "SR-DI-BPM-063:X", "SR-DI-BPM-064:X", "SR-DI-BPM-065:X", "SR-DI-BPM-066:X", "SR-DI-BPM-067:X", "SR-DI-BPM-071:X", "SR-DI-BPM-072:X", "SR-DI-BPM-073:X", "SR-DI-BPM-074:X", "SR-DI-BPM-075:X", "SR-DI-BPM-076:X", "SR-DI-BPM-077:X", "SR-DI-BPM-081:X", "SR-DI-BPM-082:X", "SR-DI-BPM-083:X", "SR-DI-BPM-084:X", "SR-DI-BPM-085:X", "SR-DI-BPM-086:X", "SR-DI-BPM-087:X", "SR-DI-BPM-091:X", "SR-DI-BPM-092:X", "SR-DI-BPM-093:X", "SR-DI-BPM-094:X", "SR-DI-BPM-095:X", "SR-DI-BPM-096:X", "SR-DI-BPM-097:X", "SR-DI-BPM-101:X", "SR-DI-BPM-102:X", "SR-DI-BPM-103:X", "SR-DI-BPM-104:X", "SR-DI-BPM-105:X", "SR-DI-BPM-106:X", "SR-DI-BPM-107:X", "SR-DI-BPM-111:X", "SR-DI-BPM-112:X", "SR-DI-BPM-113:X", "SR-DI-BPM-114:X", "SR-DI-BPM-115:X", "SR-DI-BPM-116:X", "SR-DI-BPM-117:X", "SR-DI-BPM-121:X", "SR-DI-BPM-122:X", "SR-DI-BPM-123:X", "SR-DI-BPM-124:X", "SR-DI-BPM-125:X", "SR-DI-BPM-126:X", "SR-DI-BPM-127:X", "SR-DI-BPM-128:X", "SR-DI-BPM-130:X", "SR-DI-BPM-131:X", "SR-DI-BPM-132:X", "SR-DI-BPM-133:X", "SR-DI-BPM-134:X", "SR-DI-BPM-135:X", "SR-DI-BPM-136:X", "SR-DI-BPM-137:X", "SR-DI-BPM-141:X", "SR-DI-BPM-142:X", "SR-DI-BPM-143:X", "SR-DI-BPM-144:X", "SR-DI-BPM-145:X", "SR-DI-BPM-146:X", "SR-DI-BPM-147:X", "SR-DI-BPM-151:X", "SR-DI-BPM-152:X", "SR-DI-BPM-153:X", "SR-DI-BPM-154:X", "SR-DI-BPM-155:X", "SR-DI-BPM-156:X", "SR-DI-BPM-157:X", "SR-DI-BPM-161:X", "SR-DI-BPM-162:X", "SR-DI-BPM-163:X", "SR-DI-BPM-164:X", "SR-DI-BPM-165:X", "SR-DI-BPM-166:X", "SR-DI-BPM-167:X", "SR-DI-BPM-171:X", "SR-DI-BPM-172:X", "SR-DI-BPM-173:X", "SR-DI-BPM-174:X", "SR-DI-BPM-175:X", "SR-DI-BPM-176:X", "SR-DI-BPM-177:X", "SR-DI-BPM-181:X", "SR-DI-BPM-182:X", "SR-DI-BPM-183:X", "SR-DI-BPM-184:X", "SR-DI-BPM-185:X", "SR-DI-BPM-186:X", "SR-DI-BPM-187:X", "SR-DI-BPM-191:X", "SR-DI-BPM-192:X", "SR-DI-BPM-193:X", "SR-DI-BPM-194:X", "SR-DI-BPM-195:X", "SR-DI-BPM-196:X", "SR-DI-BPM-197:X", "SR-DI-BPM-201:X", "SR-DI-BPM-202:X", "SR-DI-BPM-203:X", "SR-DI-BPM-204:X", "SR-DI-BPM-205:X", "SR-DI-BPM-206:X", "SR-DI-BPM-207:X", "SR-DI-BPM-208:X", "SR-DI-BPM-210:X", "SR-DI-BPM-211:X", "SR-DI-BPM-212:X", "SR-DI-BPM-213:X", "SR-DI-BPM-214:X", "SR-DI-BPM-215:X", "SR-DI-BPM-216:X", "SR-DI-BPM-217:X", "SR-DI-BPM-221:X", "SR-DI-BPM-222:X", "SR-DI-BPM-223:X", "SR-DI-BPM-224:X", "SR-DI-BPM-225:X", "SR-DI-BPM-226:X", "SR-DI-BPM-227:X", "SR-DI-BPM-231:X", "SR-DI-BPM-232:X", "SR-DI-BPM-233:X", "SR-DI-BPM-234:X", "SR-DI-BPM-235:X", "SR-DI-BPM-236:X", "SR-DI-BPM-237:X", "SR-DI-BPM-241:X", "SR-DI-BPM-242:X", "SR-DI-BPM-243:X", "SR-DI-BPM-244:X", "SR-DI-BPM-245:X", "SR-DI-BPM-246:X", "SR-DI-BPM-247:X"]  # sorted BPMX_174
    w360 = string[] ["BL-05A:HutchA_Enable", "BL-09A:HutchA_Enable", "BL-21A:HutchA_Enable", "BL-23A:HutchA_Enable", "BL-25A:HutchA_Enable", "BL-41A:HutchA_Enable", "BL-45A:HutchA_Enable"]  # Hutch enable
    w379 = string[] ["CPCI03-adl7452-0:doBank0Ch5", "CPCI05-adl7452-0:doBank0Ch5", "CPCI11-adl7452-0:doBank0Ch5", "CPCI12-adl7452-0:doBank0Ch5", "CPCI13-adl7452-0:doBank0Ch5", "CPCI21-adl7452-0:doBank0Ch5", "CPCI23-adl7452-0:doBank0Ch5"]  # FE enable
    (unwired) 1 ("index")
    w456 = 578.303 ("y")
    w461 = 1.202 ("y")
    # "D:\\LOG運轉紀錄\\2016"
    # "45"
    # "41"
    # "25"
    # "23"
    # "21"
    # "09"
    # "05"
    # "0為"
    # "05\n09\n21\n23\n25\n41\n45"
    # "gapMotorOff"
    n28 = disable-structure shown="Disabled" {
      frame Disabled {
        n29 = call-poly <userlib>:"CaLabGet.vi"("PV Name"="TI-INJ-PROC:getTrig-LI-EGUN") -> ("1rst Value (string)"=w621:string)  [unwired: 8 in, 6 out]
        n30 = Equal?(x="1" ("1rst Value (string)"), y=w621) -> (x = y?=w619:bool)
        n31 = case shown="True" w619 {
          frame False {
          }
          frame True {
            n32 = local read item#-1() -> (→"date (last Gun ON)")
            n33 = local read item#-1() -> (→"time string (last Gun ON)")
          }
        }
      }
      frame Enabled {
      }
    }
    n34 = event shown="[3] \"Save Button\": Value Change" {
      selector: _ -> [_ _ _ _]
      dyn-events: _ -> [_ _ _ _]
      timeout: 233 -> [_ _ _ _]
      tunnel: [_ w484 _ _] -> w46
      tunnel: [w482 w483 w485 w522] -> w45
      tunnel: w44 -> [w482 w483 w485 _]
      event Timeout {
        n35 = event-data() -> ()  [unwired: 1 in, 3 out]
      }
      event "stop": Value Change {
        n36 = event-data() -> ("NewVal"=w484:bool)  [unwired: 1 in, 3 out]
      }
      event "Open Button": Value Change {
        n37 = event-data() -> ()  [unwired: 1 in, 6 out]
        n38 = Get Date/Time In Seconds() -> (seconds since 1Jan1904=w506:timestamp)
        n39 = Format Date/Time String(time format string (%c)="%Y", seconds (now)=w506, UTC format=FALSE) -> (date/time string=w498:string)
        n40 = Format Date/Time String(time format string (%c)="%d", seconds (now)=w506, UTC format=FALSE) -> (date/time string=w489:string)
        n41 = call "to_be_2_string.vi"("string 2"=w489) -> ("substring 2"=w488:string)  [unwired: 10 in]
        n42 = Format Date/Time String(time format string (%c)="%m", seconds (now)=w506, UTC format=FALSE) -> (date/time string=w494:string)
        n43 = Concatenate Strings("D" ("磁碟位置"), ":\\LOG運轉紀錄\\", w498, "\\", w494, "\\", w488) -> (w486:string)
        n44 = String To Path(string=w486) -> (path=w502:path)
        n45 = call <vilib>:"Check if File or Folder Exists.vi"("path"=w502) -> ("error out"=w504:errorcluster, "file or folder exists?"=w490:bool, "dup path"=w503:path)  [unwired: 8 in]
        n46 = case shown="False" w490 {
          tunnel: w503 -> [w513 w515]
          tunnel: w504 -> [w512 w514]
          tunnel: [w511 w515] -> _
          tunnel: [w510 w514] -> w487
          frame False {
            n47 = Create Folder(path (use dialog)=w513, error in=w512) -> (created path=w511:path, error out=w510:errorcluster)  [unwired: 1 in, 1 out]
          }
          frame True {
          }
        }
        n48 = Concatenate Strings("explorer ", w486) -> (w508:string)
        n49 = call <vilib>:"System Exec.vi"("wait until completion? (T)"=FALSE, "error in (no error)"=w487, "command line"=w508) -> ()  [unwired: 5 in, 4 out]
      }
      event "Save Button": Value Change {
        n50 = event-data() -> ()  [unwired: 1 in, 1 out]
        n51 = flat-sequence {
          tunnel: [w525] -> w520
          tunnel: [w524] -> w519
          tunnel: [w523] -> w518
          tunnel: [w565] -> w521
          tunnel: w520 -> [w565]
          tunnel: w519 -> [w563]
          tunnel: w518 -> [w564]
          tunnel: [w564] -> w517
          tunnel: [w563] -> w516
          tunnel: [w572] -> w522
          tunnel: w521 -> [w572]
          tunnel: w517 -> [w568]
          tunnel: w516 -> [w567]
          frame #0 {
            n52 = Multiply(x=3600.0 ("y"), y="last ? Hrs") -> (x*y=w533:dbl)
            n53 = Get Date/Time In Seconds() -> (seconds since 1Jan1904=w523:timestamp)
            n54 = Subtract(x=w523, y=w533) -> (x-y=w524:timestamp)
            n55 = call "TimeToString.vi"("Time Stamp Control"=w523) -> ("result string"=w531:string)
            n56 = call "TimeToString.vi"("Time Stamp Control"=w524) -> ("result string"=w532:string)
            n57 = call <vilib>:"Application Directory.vi"() -> ("Application Directory"=w530:path)
            n58 = Build Path(base path=w530, name or relative path="DSN\\172-18-0-32.dsn") -> (appended path=w528:path)
            n59 = call-poly <vilib>:"DB Tools Open Connection.vi"("connection information"=w528) -> ("error out"=w540:errorcluster, "connection reference"=w541:T2)  [unwired: 7 in]
            n60 = Concatenate Strings("SELECT  float_val , smpl_time\nFROM sample \nwhere  channel_id = 104 and smpl_time between '" ("result string"), w532, "' ::timestamp and '" ("result string"), w531, "' ::timestamp" ("result string")) -> (w556:string)
            n61 = call-poly <vilib>:"DB Tools Execute Query.vi"("error in (no error)"=w540, "SQL query"=w556, "connection reference"=w541) -> ("error out"=w543:errorcluster, "recordset reference"=w542:T3)  [unwired: 5 in]
            n62 = call-poly <vilib>:"DB Tools Fetch Recordset Data.vi"("error in (no error)"=w543, "recordset reference"=w542) -> ("error out"=w545:errorcluster, "recordset data"=w548:variant[][], "recordset reference out"=w544:T3)  [unwired: 3 in]
            n63 = call-poly <vilib>:"DB Tools Free Object.vi"("error in (no error)"=w545, "recordset reference"=w544) -> ("error out"=w547:errorcluster, "connection reference"=w546:T2)  [unwired: 8 in]
            n64 = Variant To Data(type=string[][] [], Variant=w548) -> (data=w550:string[][])  [unwired: 1 in, 1 out]
            n65 = call <vilib>:"DB Tools Close Connection.vi"("error in (no error)"=w547, "connection reference"=w546) -> ("error out"=→"error out 2":errorcluster)  [unwired: 5 in]
            n66 = Transpose 2D Array(2D array=w550) -> (transposed array=w552:string[][])
            n67 = Index Array(array=w552, index (row) #1=0 ("index (row)"), index (row) #2=1 ("index (row)")) -> (element #1=w538:string[], element #2=w535:string[])  [unwired: 2 in]
            n68 = for {
              tunnel: w535 -> [w559] mode=indexing
              tunnel: [w558] -> w537 mode=indexing
              n69 = Scan From String "Scan From String"(format string="%<%Y/%m/%d %p %I:%M:%S>T", input string=w559, initial scan location=u32 0, default 1=timestamp(-73814400 s since 1904-01-01)) -> (output 1=w562:timestamp)  [unwired: 1 in, 3 out]
              n70 = To Double Precision Float(number=w562) -> (double precision float=w558:dbl)
            }
            n71 = Fract/Exp String To Number(string=w538) -> (number=w536:dbl[])  [unwired: 3 in, 1 out]
            n72 = Bundle(w537, w536) -> (w525:cluster{dbl[], dbl[]})  [unwired: 1 in]
          }
          frame #1 {
            n73 = Wait (ms)(milliseconds to wait=u32 300) -> ()  [unwired: 1 out]
          }
          frame #2 {
            n74 = Get Date/Time In Seconds() -> (seconds since 1Jan1904=w575:timestamp)
            n75 = Format Date/Time String(time format string (%c)="%Y", seconds (now)=w575, UTC format=FALSE) -> (date/time string=w594:string)
            n76 = Format Date/Time String(time format string (%c)="%d", seconds (now)=w575, UTC format=FALSE) -> (date/time string=w603:string)
            n77 = call "to_be_2_string.vi"("string 2"=w603) -> ("substring 2"=w604:string)  [unwired: 10 in]
            n78 = Format Date/Time String(time format string (%c)="%m", seconds (now)=w575, UTC format=FALSE) -> (date/time string=w598:string)
            n79 = Format Date/Time String(time format string (%c)="%Y%m%d%H%M%S", seconds (now)=w575) -> (date/time string=w582:string)  [unwired: 1 in]
            n80 = Concatenate Strings("D" ("磁碟位置"), ":\\LOG運轉紀錄\\", w594, "\\", w598, "\\", w604) -> (w587:string)
            n81 = String To Path(string=w587) -> (path=w590:path)
            n82 = call <vilib>:"Check if File or Folder Exists.vi"("path"=w590) -> ("error out"=w588:errorcluster, "file or folder exists?"=w602:bool, "dup path"=w589:path)  [unwired: 8 in]
            n83 = invoke on="Cluster" class="Clust (strict)" method="Get Image"() -> ("image data"=w573:T5)  [unwired: 6 in, 5 out]
            n84 = case shown="False" w602 {
              tunnel: w589 -> [w608 w610]
              tunnel: w588 -> [w607 w609]
              tunnel: [w606 w610] -> w574
              tunnel: [w605 w609] -> _
              frame False {
                n85 = Create Folder(path (use dialog)=w608, error in=w607) -> (created path=w606:path, error out=w605:errorcluster)  [unwired: 1 in, 1 out]
              }
              frame True {
              }
            }
            n86 = Path To String(path=w574) -> (string=w586:string)
            n87 = control-ref of="BeamCurrent History"() -> (w571:refnum<vi>)
            n88 = To Double Precision Float(number=w568) -> (double precision float=w570:dbl)
            n89 = To Double Precision Float(number=w567) -> (double precision float=w569:dbl)
            n90 = Concatenate Strings(w586, "\\" ("string"), w582) -> (w576:string)
            n91 = property on="Property Node" class="XYGraph (strict)"(reference=w571, "XScale.Maximum"=w570, "XScale.Minimum"=w569) -> ()  [unwired: 1 in, 2 out]
            n92 = Concatenate Strings(w576, ".jpg" ("file format")) -> (w577:string)
            n93 = String To Path(string=w577) -> (path=w581:path)
            n94 = call <vilib>:"Write JPEG File.vi"("quality (80)"=100, "image data"=w573, "path to JPEG file"=w581) -> ("error out"=→"error out 3":errorcluster)  [unwired: 7 in, 1 out]
          }
        }
      }
    }
    n95 = disable-structure shown="Disabled" {
      frame Disabled {
        n96 = Bundle By Name(cluster=T4 {"SR Fill Pattern"=array[864 elements], "Beam Current(mA"=301.91562200000004, "Beam Lifetime(min)"=669.1065769463743, "Beamsize X(um)"=55.54579477590784, "Beamsize Y(um)"=33.648665625479325, "Tune X(from BPM)"=0.1399, "Tune Y(from BPM)"=0.14, "Mode"="Top-Up", "NuX(from BBF) "=0.16718639681347974, "NuY(from BBF)"=0.25219386232318686, "IU22-23gap(R)"=11.0, "IU22-05gap(R)"=7.558, "IU22-05M"=TRUE, "IU22A-09gap(R)"=8.075, "IU22A-09M"=TRUE, "IU22B-09gap(R)"=40.001, "IU22B-09M"=FALSE, "IUT22-21gap(R)"=7.0, "IUT22-21M"=TRUE, "IU22-23M"=TRUE, "IU22A-25gap(R)"=8.18, "IU22A-25M"=TRUE, "IU22B-25gap(R)"=40.0, "IU22B-25M"=FALSE, "EPU48A-41gap(R)"=64.99985000000001, "EPU48A-41gM"=TRUE, "EPU48B-41gap(R)"=65.00399999999999, "EPU48B-41gM"=FALSE, "EPU46-45gap(R)"=45.00005, "EPU46-45gM"=TRUE, "EPU48A-41phase(R)"=0.0001, "EPU48B-41phase(R)"=0.00055, "EPU46-45phase(R)"=0.0, "Grid volt.(V)(S)"=33.0, "Gun mode"="MBM", "Mod.3 HV(kV)(S)"=35.800000000000026, "SR"="SR_DMB_2016_1102_1124LOCO.data", "BR"="Booster_JT_2016_1005_1200.data", "Linac"="Linac2016_1005_0935.data", "LTB"="LTB_JT_2016_1005_1200.data", "BTS"="BTS_2016_1116_1020.data", "RF2 remote"=TRUE, "RF2 OP mode"=TRUE, "RF2 phase.(S)"=-56.70000000000001, "RF Freq.(s)"=499654660.62238467, "RF2 gap volt.(S)"=1400.0, "RF3 remote"=TRUE, "RF3 OP mode"=TRUE, "RF3 phase.(S)"=160.0, "RF3 gap volt.(S)"=1400.0, "BBF V"=TRUE, "BBF H"=TRUE, "BR ext. kicker1(kV)"=18.266, "BR ext. kicker2(kV)"=18.26600000000001, "BR ext. sep.1(V)"=318.8444, "BR ext. sep.2(V)"=444.5, "BR inj. sep.(V)"=105.2, "BR inj. kicker(kV)"=16.40000000000001, "SR kicker4(kV)"=8.27, "SR kicker3(kV)"=8.315, "SR kicker2(kV)"=8.325, "SR kicker1(kV)"=8.4, "SR inj. sep.2(V)"=417.0, "SR inj. sep.1(V)"=419.3416, "Bucket Start"=100.0, "Bucket Last"=630.0, "Bucket Step"=10.0, "Orbit ILK(P)"=TRUE, "IU22-05 Hutch Enable"=TRUE, "IU22A-09M Hutch Enable"=TRUE, "IUT22-21M Hutch Enable"=TRUE, "IU22-23M Hutch Enable"=FALSE, "IU22A-25M Hutch Enable"=TRUE, "EPU48A-41M Hutch Enable"=FALSE, "EPU46-45M Hutch Enable"=TRUE, "EPU46-45 FE Enable"=TRUE, "EPU48A-41 FE Enable"=FALSE, "IU22A-25 FE Enable"=TRUE, "IU22-23 FE Enable"=FALSE, "IUT22-21 FE Enable"=TRUE, "IU22A-09 FE Enable"=TRUE, "IU22-05 FE Enable"=TRUE, "EPU48A-41pM"=TRUE, "EPU48B-41pM"=FALSE, "EPU46-45pM"=FALSE, "Gun volt.(V)(S)"=23.5, "Width count"=30.0, "2ns step"=0.0, "10ps delay"=100.0, "phase shifter"=130.00060000000002, "Taper"=-1.0899999999999999, "05XBPMX 1"=115.877, "09XBPMX 1"=471.421, "21XBPMX 1"=612.331, "23XBPMX 1"=-46.736000000000004, "25XBPMX 1"=462.29900000000004, "41XBPMX 1"=364.139, "45XBPMX 1"=-164.196, "05XBPMY 1"=-62.875, "09XBPMY 1"=-23.034, "21XBPMY 1"=-27.449, "23XBPMY 1"=-89.72200000000001, "25XBPMY 1"=459.291, "41XBPMY 1"=-111.624, "45XBPMY 1"=-57.689, "FOFB H"="On", "FOFB V"="On", "time string"="21:36:25", "date"="2016/11/21", "date (last kicker ON)"="wait to fire", "time string (last kicker ON)"="", "BPMX Graph"={[1, 2, 3, 4, 5, 6, 7, 8, 9, 10, 11, 12, 13, 14, 15, 16, 17, 18, 19, 20, 21, 22, 23, 24, 25, 26, 27, 28, 29, 30, 31, 32, 33, 34, 35, 36, 37, 38, 39, 40, 41, 42, 43, 44, 45, 46, 47, 48, 49, 50, 51, 52, 53, 54, 55, 56, 57, 58, 59, 60, 61, 62, 63, 64, 65, 66, 67, 68, 69, 70, 71, 72, 73, 74, 75, 76, 77, 78, 79, 80, 81, 82, 83, 84, 85, 86, 87, 88, 89, 90, 91, 92, 93, 94, 95, 96, 97, 98, 99, 100, 101, 102, 103, 104, 105, 106, 107, 108, 109, 110, 111, 112, 113, 114, 115, 116, 117, 118, 119, 120, 121, 122, 123, 124, 125, 126, 127, 128, 129, 130, 131, 132, 133, 134, 135, 136, 137, 138, 139, 140, 141, 142, 143, 144, 145, 146, 147, 148, 149, 150, 151, 152, 153, 154, 155, 156, 157, 158, 159, 160, 161, 162, 163, 164, 165, 166, 167, 168, 169, 170, 171, 172, 173, 174], "1rst Value (number)"=[-31.198, -3.303, -73.172, -2.032, 86.386, -75.851, 71.519, -46.03, 6.824, -37.804, 68.275, -4.672, -223.404, -16.867, -6.964, -259.448, -62.697, 1.8880000000000001, 75.267, -92.668, 86.714, -30.843, 12.767, -107.398, -44.436, 161.126, 208.922, 211.488, -27.247, 79.489, 826.962, 470.705, -115.522, -41.497, 159.486, -54.261, -0.64, 42.641, -2.466, -143.394, -24.785, 138.912, -65.805, 42.325, 32.891, -7.298, -96.724, -31.725, 98.531, -80.64, 64.163, 94.83, -44.03, -163.192, 50.589, 46.669000000000004, -87.508, 78.479, 31.618000000000002, -17.077, -125.32600000000001, -3.845, 98.34100000000001, -39.679, 50.247, -58.208, 40.297000000000004, -69.857, 42.548, -19.403, -211.0, -9.082, -322.597, -233.847, -140.75, 97.087, -15.869, -29.053, 59.46, -115.316, 70.896, -60.685, 33.715, 12.09, -520.422, -138.423, -302.753, 79.862, 120.014, 122.671, -55.812, 27.084, 39.115, -138.936, 156.631, 53.777, -72.647, -52.588, 16.002, 45.197, -117.489, 121.709, 27.952, -31.609, -113.58500000000001, 45.019, 55.136, -130.553, 138.93200000000002, 35.998, -30.631, -96.529, -7.589, 100.395, -93.919, 40.569, 79.538, -68.044, -134.578, 2.52, 84.539, -59.166000000000004, 42.576, 34.657000000000004, -15.805, -52.158, 18.484, 4.346, -157.404, 182.672, 202.518, -164.868, -53.871, 8.066, -9.738, -55.594, 92.623, -13.785, 11.587, -60.627, -47.704, 65.516, 57.924, 148.347, -201.348, -302.753, 189.117, 72.681, -134.928, 39.791000000000004, 45.938, -49.072, 54.473, 28.991, -20.657, -80.283, -20.264, 106.907, -121.271, 150.281, -2.243, -11.844, -122.82300000000001, 0.973, 114.186, -107.94, 95.485, 40.314, -36.956, -134.537, 16.196, 91.88, -35.505, -0.018000000000000002]}, "BPMY Graph"={[1, 2, 3, 4, 5, 6, 7, 8, 9, 10, 11, 12, 13, 14, 15, 16, 17, 18, 19, 20, 21, 22, 23, 24, 25, 26, 27, 28, 29, 30, 31, 32, 33, 34, 35, 36, 37, 38, 39, 40, 41, 42, 43, 44, 45, 46, 47, 48, 49, 50, 51, 52, 53, 54, 55, 56, 57, 58, 59, 60, 61, 62, 63, 64, 65, 66, 67, 68, 69, 70, 71, 72, 73, 74, 75, 76, 77, 78, 79, 80, 81, 82, 83, 84, 85, 86, 87, 88, 89, 90, 91, 92, 93, 94, 95, 96, 97, 98, 99, 100, 101, 102, 103, 104, 105, 106, 107, 108, 109, 110, 111, 112, 113, 114, 115, 116, 117, 118, 119, 120, 121, 122, 123, 124, 125, 126, 127, 128, 129, 130, 131, 132, 133, 134, 135, 136, 137, 138, 139, 140, 141, 142, 143, 144, 145, 146, 147, 148, 149, 150, 151, 152, 153, 154, 155, 156, 157, 158, 159, 160, 161, 162, 163, 164, 165, 166, 167, 168, 169, 170, 171, 172, 173, 174], "1rst Value (number)"=[-99.743, 2.851, -30.024, 83.777, -46.733000000000004, -39.889, 2.349, -4.944, 17.022000000000002, 9.824, 11.632, 41.188, -13.992, 13.911, -6.211, 53.857, -48.993, -32.789, -6.3740000000000006, -62.867000000000004, -8.332, 72.09400000000001, -75.398, 53.283, 63.008, -2.23, 43.024, 32.073, -246.641, -93.162, 456.41700000000003, 88.299, 58.803000000000004, 1.7590000000000001, 35.664, 6.575, 18.59, -30.439, 11.254, -28.256, -62.707, -4.503, 1.31, -21.571, 34.77, -8.876, 31.237000000000002, 25.402, 2.726, 20.655, -7.845, -1.443, -31.935000000000002, -16.981, 13.022, 17.515, -82.867, 61.285000000000004, -57.573, 110.363, -27.753, 28.322, -9.241, 53.929, -25.816, 24.231, -57.876, -11.578, 32.087, -70.84, 64.43, 9.409, -157.639, -57.0, 39.267, 30.23, 18.993000000000002, -33.97, 26.195, -10.585, -17.617, -18.667, 31.615000000000002, -25.437, 29.564, 13.537, 6.728, 163.38400000000001, 106.51, -70.056, 12.874, -4.125, -10.855, -21.856, 1.947, 8.096, 11.402000000000001, 5.761, 41.929, -8.752, 18.634, 7.553, -40.034, 39.183, -25.067, -32.557, 5.393, -17.564, -1.614, 20.498, -14.818, 10.313, 35.254, -35.886, 58.359, -36.56, -20.354, 7.593, -21.256, -8.001, -16.79, 10.18, -16.327, 20.416, -10.539, 19.944, -6.801, 13.068, -13.644, 3.468, -0.983, -17.6, 6.785, -26.101, -11.52, 61.191, -32.777, 13.536, 4.026, -14.682, 52.057, -53.883, 27.118000000000002, 31.672, 79.62, 17.715, 15.693, 113.157, -57.095, 14.214, -4.787, -11.148, -3.157, -6.251, -0.764, 3.563, 7.3500000000000005, 10.779, 21.129, 11.36, 7.771, -14.787, -13.278, 0.279, -13.516, -62.422000000000004, -13.389000000000001, 80.56400000000001, -108.465, 69.885, 30.116, 21.421, 32.779, -10.527000000000001]}, "Radio Buttons 2"=enum."absolute", "09XBPMX 2"="", "09XBPMY 2"="", "05XBPMY 2"="", "05XBPMX 2"="", "21XBPMY 2"="", "21XBPMX 2"="", "23XBPMY 2"="", "23XBPMX 2"="", "25XBPMY 2"="", "25XBPMX 2"="", "41XBPMY 2"="", "41XBPMX 2"="", "45XBPMX 2"="", "45XBPMY 2"="", "05 mode"="", "09A mode"="", "09B mode"="", "21 mode"="", "23 mode"="", "25A mode"="", "25B mode"="", "41A mode"="", "41B mode"="", "46 mode"="", "BeamCurrent History"={"BPM NO.  1_172"=[3587880327.0, 3587880337.0, 3587880347.0, 3587880357.0, 3587880367.0, 3587880377.0, 3587880388.0, 3587880398.0, 3587880408.0, 3587880417.0, 3587880427.0, 3587880437.0, 3587880447.0, 3587880457.0, 3587880467.0, 3587880477.0, 3587880487.0, 3587880497.0, 3587880507.0, 3587880517.0, 3587880527.0, 3587880537.0, 3587880547.0, 3587880557.0, 3587880567.0, 3587880577.0, 3587880587.0, 3587880597.0, 3587880607.0, 3587880617.0, 3587880627.0, 3587880637.0, 3587880647.0, 3587880657.0, 3587880667.0, 3587880677.0, 3587880687.0, 3587880697.0, 3587880707.0, 3587880717.0, 3587880727.0, 3587880737.0, 3587880747.0, 3587880757.0, 3587880767.0, 3587880777.0, 3587880787.0, 3587880797.0, 3587880807.0, 3587880817.0, 3587880827.0, 3587880837.0, 3587880847.0, 3587880857.0, 3587880867.0, 3587880877.0, 3587880887.0, 3587880897.0, 3587880907.0, 3587880917.0], [279.8706, 279.6878, 279.5138, 279.3326, 279.1537, 278.9744, 280.1668, 279.9874, 279.8097, 279.6281, 279.4484, 279.2734, 279.0933, 279.9395, 280.0027, 279.8235, 279.642, 279.4661, 279.2873, 279.1089, 279.6484, 280.0044, 279.8243, 279.6482, 279.4694, 279.2899, 279.1109, 279.5519, 279.9906, 279.8127, 279.6339, 279.4608, 279.2828, 279.104, 279.6982, 279.9463, 279.7671, 279.5915, 279.4126, 279.2368, 279.0606, 280.1311, 279.9543, 279.7767, 279.6011, 279.4247, 279.2452, 279.0726, 280.2098, 280.0333, 279.8566, 279.6814, 279.5039, 279.3286, 279.1559, 278.9767, 280.1638, 279.9891, 279.8148, 279.6383]}, "SR Beam Current in Last           Hrs"=12.0} ("Cluster")) -> (w479:T4)  [unwired: 1 in]
        n97 = local write "Cluster"(w479) -> ()
      }
      frame Enabled {
      }
    }
    n98 = call-poly <userlib>:"CaLabGet.vi"("PV Names"=string[] ["FE-DI-XBPM-051:signals:sa.X", "FE-DI-XBPM-051:signals:sa.Y", "FE-DI-XBPM-091:SA:SA_X_MONITOR", "FE-DI-XBPM-091:SA:SA_Y_MONITOR", "FE-DI-XBPM-211:SA:SA_X_MONITOR", "FE-DI-XBPM-211:SA:SA_Y_MONITOR", "FE-DI-XBPM-231:SA:SA_X_MONITOR", "FE-DI-XBPM-231:SA:SA_Y_MONITOR", "FE-DI-XBPM-251:SA:SA_X_MONITOR", "FE-DI-XBPM-251:SA:SA_Y_MONITOR", "FE-DI-XBPM-411:SA:SA_X_MONITOR", "FE-DI-XBPM-411:SA:SA_Y_MONITOR", "FE-DI-XBPM-451:SA:SA_X_MONITOR", "FE-DI-XBPM-451:SA:SA_Y_MONITOR", "FE-DI-XBPM-052:signals:sa.X", "FE-DI-XBPM-052:signals:sa.Y", "FE-DI-XBPM-092:SA:SA_X_MONITOR", "FE-DI-XBPM-092:SA:SA_Y_MONITOR", "FE-DI-XBPM-212:SA:SA_X_MONITOR", "FE-DI-XBPM-212:SA:SA_Y_MONITOR", "FE-DI-XBPM-232:SA:SA_X_MONITOR", "FE-DI-XBPM-232:SA:SA_Y_MONITOR", "FE-DI-XBPM-252:SA:SA_X_MONITOR", "FE-DI-XBPM-252:SA:SA_Y_MONITOR", "FE-DI-XBPM-412:SA:SA_X_MONITOR", "FE-DI-XBPM-412:SA:SA_Y_MONITOR", "FE-DI-XBPM-452:SA:SA_X_MONITOR", "FE-DI-XBPM-452:SA:SA_Y_MONITOR"] ("appended array")) -> ("1rst Value (number)"=w327:dbl[])  [unwired: 8 in, 6 out]
    n99 = Multiply(x=w327, y=0.001) -> (x*y=w326:dbl[])
    "Value Array (number) 7" <- w326
    n100 = disable-structure shown="Disabled" {
      frame Disabled {
        n101 = To Long Integer() -> (32bit integer=w661:i32)  [unwired: 1 in]
        n102 = case shown="1" w661 {
          tunnel: ["Decay" "Top-Up"] -> _
          frame 0, Default {
          }
          frame 1 {
          }
        }
      }
      frame Enabled {
      }
    }
    n103 = Index Array(array=w326, index #1=0 ("index"), index #2=1 ("index"), index #3=2 ("index"), index #4=3 ("index"), index #5=4 ("index"), index #6=5 ("index"), index #7=6 ("index"), index #8=7 ("index"), index #9=8 ("index"), index #10=9 ("index"), index #11=10 ("index"), index #12=11 ("index"), index #13=12 ("index"), index #14=13 ("index"), index #15=14 ("index"), index #16=15 ("index"), index #17=16 ("index"), index #18=17 ("index"), index #19=18 ("index"), index #20=19 ("index"), index #21=20 ("index"), index #22=21 ("index"), index #23=22 ("index"), index #24=23 ("index"), index #25=24 ("index"), index #26=25 ("index"), index #27=26 ("index"), index #28=27 ("index")) -> (element #1=w242:dbl, element #2=w235:dbl, element #3=w241:dbl, element #4=w234:dbl, element #5=w240:dbl, element #6=w233:dbl, element #7=w239:dbl, element #8=w232:dbl, element #9=w238:dbl, element #10=w231:dbl, element #11=w237:dbl, element #12=w230:dbl, element #13=w236:dbl, element #14=w229:dbl, element #15=w128:dbl, element #16=w127:dbl, element #17=w126:dbl, element #18=w125:dbl, element #19=w116:dbl, element #20=w115:dbl, element #21=w110:dbl, element #22=w109:dbl, element #23=w108:dbl, element #24=w107:dbl, element #25=w76:dbl, element #26=w75:dbl, element #27=w74:dbl, element #28=w73:dbl)
    n104 = call-poly <userlib>:"CaLabGet.vi"("PV Names"=string[] ["LI-ES-CPS-01:PULSEMODE", "LI-ES-BPS-01:SETU:GRID", "LI-ES-BPS-01:SETU:MBM", "LI-ES-BPS-01:SETU:SBM", "LI-RF-HVP-31:SET:U", "CPCITM-TI-EVRTG:Pulse6DelaySet", "CPCITM-TI-EVRTG:Pulse7DelaySet", "CPCITM-TI-EVRTG:Pulse6WidthSet", "CPCITM-TI-EVRTG:Pulse7WidthSet", "CPCITM-TI-EVRTG:GTX6CtrlGTXPHSet", "CPCITM-TI-EVRTG:GTX7CtrlGTXPHSet", "CPCITM-TI-EVRTG:GTX6DlySet", "CPCITM-TI-EVRTG:GTX7DlySet"]) -> ("1rst Value (string)"=w389:string[], "1rst Value (number)"=w440:dbl[])  [unwired: 8 in, 5 out]
    "Value Array (number) 3" <- w440
    "1rst Value (string) 2" <- w389
    n105 = call-poly <userlib>:"CaLabGet.vi"("PV Names"=string[] ["BR-PS-INJ-SE:setHV", "BR-PS-INJ-KI:setHV", "BR-PS-EXT-K1:setHV", "BR-PS-EXT-K2:setHV", "BR-PS-EXT-SE1:setHV", "BR-PS-EXT-SE2:setHV", "SR-PS-INJ-SE1:setHV", "SR-PS-INJ-SE2:setHV", "SR-PS-INJ-K1:setHV", "SR-PS-INJ-K2:setHV", "SR-PS-INJ-K3:setHV", "SR-PS-INJ-K4:setHV"]) -> ("1rst Value (number)"=w442:dbl[])  [unwired: 8 in, 6 out]
    "Value Array (number) 2" <- w442
    n106 = call-poly <userlib>:"CaLabGet.vi"("PV Names"=string[] ["SR-RF-MSG:setFreq", "SR-RF2-LLRF:local", "SR-RF2-LLRF:getOperationMode", "SR-RF2-LLRF:getGapVoltage", "SR-RF2-LLRF:setGapVoltage", "SR-RF2-LLRF:setStationPhase", "SR-RF3-LLRF:local", "SR-RF3-LLRF:getOperationMode", "SR-RF3-LLRF:getGapVoltage", "SR-RF3-LLRF:setGapVoltage", "SR-RF3-LLRF:setStationPhase"]) -> ("1rst Value (number)"=w415:dbl[])  [unwired: 8 in, 6 out]
    "Value Array (number) 4" <- w415
    n107 = call-poly <userlib>:"CaLabGet.vi"("PV Names"=string[] ["SR-DI-FP:CurrentBuffer"]) -> ("Value Array (number)"=w397:dbl[][])  [unwired: 8 in, 6 out]
    n108 = call-poly <userlib>:"CaLabGet.vi"("PV Names"=string[] ["TI-INJ-PROC:TopupHiLowStart", "SR-DI-DCCT:BeamCurrent", "SR-DI-DCCT:BeamLifetime", "SR-DI-XPC-40:SigmaX", "SR-DI-XPC-40:SigmaY", "SR-DI-TUNE:nux", "SR-DI-TUNE:nuy", "IGPF:TPSX:SRAM:VEC:PEAKFREQ2", "IGPF:TPSY:SRAM:VEC:PEAKFREQ2", "TI-INJ-PROC:setBucketAddressStart", "TI-INJ-PROC:setBucketAddressLast", "TI-INJ-PROC:setBucketAddressStep"]) -> ("1rst Value (number)"=w476:dbl[])  [unwired: 8 in, 6 out]
    "Value Array (number)" <- w476
    n109 = call-poly <userlib>:"CaLabGet.vi"("PV Names"=string[] ["LI:restoreFilename", "LTB:restoreFilename", "BR:restoreFilename", "BTS:restoreFilename", "SR:restoreFilename"]) -> ("1rst Value (string)"=w399:string[])  [unwired: 8 in, 6 out]
    "1rst Value (string)" <- w399
    n110 = Index Array(array=w389, index=0) -> (element=w387:string)
    n111 = Index Array(array=w440, index #1=0 ("index"), index #2=1 ("index"), index #3=2 ("index"), index #4=3 ("index"), index #5=4 ("index"), index #6=5 ("index"), index #7=6 ("index"), index #8=7 ("index"), index #9=8 ("index"), index #10=9 ("index"), index #11=10 ("index"), index #12=11 ("index"), index #13=12 ("index")) -> (element #2=w275:dbl, element #3=w391:dbl, element #4=w390:dbl, element #5=w273:dbl, element #8=w386:dbl, element #9=w385:dbl, element #10=w384:dbl, element #11=w383:dbl, element #12=w382:dbl, element #13=w381:dbl)  [unwired: 3 out]
    "MBM volt.(S)" <- w391
    "SBM volt.(S)" <- w390
    n112 = Index Array(array=w442, index #1=0 ("index"), index #2=1 ("index"), index #3=2 ("index"), index #4=3 ("index"), index #5=4 ("index"), index #6=5 ("index"), index #7=6 ("index"), index #8=7 ("index"), index #9=8 ("index"), index #10=9 ("index"), index #11=10 ("index"), index #12=11 ("index")) -> (element #1=w288:dbl, element #2=w287:dbl, element #3=w286:dbl, element #4=w285:dbl, element #5=w284:dbl, element #6=w283:dbl, element #7=w282:dbl, element #8=w281:dbl, element #9=w280:dbl, element #10=w279:dbl, element #11=w278:dbl, element #12=w277:dbl)
    n113 = Index Array(array=w415, index #1=0 ("index"), index #2=1 ("index"), index #3=2 ("index"), index #4=3 ("index"), index #5=4 ("index"), index #6=5 ("index"), index #7=6 ("index"), index #8=7 ("index"), index #9=8 ("index"), index #10=9 ("index"), index #11=10 ("index")) -> (element #1=w267:dbl, element #2=w412:dbl, element #3=w410:dbl, element #5=w188:dbl, element #6=w189:dbl, element #7=w407:dbl, element #8=w406:dbl, element #10=w263:dbl, element #11=w264:dbl)  [unwired: 2 out]
    n114 = Index Array(array=w397, index (row)=0 ("index")) -> (element=w257:dbl[])  [unwired: 1 in]
    n115 = Index Array(array=w476, index #1=0 ("index"), index #2=1 ("index"), index #3=2 ("index"), index #4=3 ("index"), index #5=4 ("index"), index #6=5 ("index"), index #7=6 ("index"), index #8=7 ("index"), index #9=8 ("index"), index #10=9 ("index"), index #11=10 ("index"), index #12=11 ("index")) -> (element #1=w474:dbl, element #2=w297:dbl, element #3=w296:dbl, element #4=w462:dbl, element #5=w460:dbl, element #6=w459:dbl, element #7=w458:dbl, element #8=w457:dbl, element #9=w455:dbl, element #10=w291:dbl, element #11=w290:dbl, element #12=w289:dbl)
    n116 = call-poly <userlib>:"CaLabGet.vi"("PV Names"=w158) -> ("1rst Value (number)"=w160:dbl[])  [unwired: 8 in, 6 out]
    n117 = Index Array(array=w399, index #1=0 ("index"), index #2=1 ("index"), index #3=2 ("index"), index #4=3 ("index"), index #5=4 ("index")) -> (element #1=w259:string, element #2=w258:string, element #3=w262:string, element #4=w261:string, element #5=w260:string)
    n118 = call-poly <userlib>:"CaLabGet.vi"("PV Names"=w360) -> ("1rst Value (string)"=w368:string[])  [unwired: 8 in, 6 out]
    n119 = To Byte Integer(number=w160) -> (8bit integer=w159:i8[])
    n120 = for {
      tunnel: w159 -> [w614] mode=indexing
      tunnel: [w611] -> w136 mode=indexing
      n121 = Number To Boolean Array(number=w614) -> (Boolean array=w613:bool[])
      n122 = Index Array(array=w613, index=0) -> (element=w611:bool)
    }
    n123 = for {
      tunnel: w368 -> [w630] mode=indexing
      tunnel: [w629] -> w369 mode=indexing
      n124 = case shown="\"Enable\"" w630 {
        tunnel: [FALSE TRUE] -> w629
        frame "Disable", Default {
        }
        frame "Enable" {
        }
      }
    }
    n125 = call-poly <userlib>:"CaLabGet.vi"("PV Names"=w379) -> ("1rst Value (string)"=w371:string[])  [unwired: 8 in, 6 out]
    n126 = call-poly <userlib>:"CaLabGet.vi"("PV Names"=string[] ["SR-ID-IU22-05:getGap", "SR-ID-IU22A-09:getGap", "SR-ID-IU22B-09:getGap", "SR-ID-IUT22-21:getGap", "SR-ID-IU22-23:getGap", "SR-ID-IU22A-25:getGap", "SR-ID-IU22B-25:getGap", "SR-ID-EPU48A-41:getGap", "SR-ID-EPU48A-41:getPhase", "SR-ID-EPU48B-41:getGap", "SR-ID-EPU48B-41:getPhase", "SR-ID-EPU46-45:getGap", "SR-ID-EPU46-45:getPhase", "SR-ID-IUT22-21:getGapTaper", "SR-ID-EPU48PS-41:getGap"]) -> ("1rst Value (number)"=w359:dbl[])  [unwired: 8 in, 6 out]
    "Value Array (number) 6" <- w359
    n127 = for {
      tunnel: w371 -> [w634] mode=indexing
      tunnel: [w633] -> w370 mode=indexing
      n128 = case shown="\"enable\"" w634 {
        tunnel: [FALSE TRUE] -> w633
        frame "disable", Default {
        }
        frame "enable" {
        }
      }
    }
    n129 = call-poly <userlib>:"CaLabGet.vi"("PV Names"=string[] ["SR-ID-IU22-05:gapMotorOff", "SR-ID-IU22A-09:gapMotorOff", "SR-ID-IU22B-09:gapMotorOff", "SR-ID-IUT22-21:gapMotorOff", "SR-ID-IU22-23:gapMotorOff", "SR-ID-IU22A-25:gapMotorOff", "SR-ID-IU22B-25:gapMotorOff", "SR-ID-EPU48A-41:gapMotorOff", "SR-ID-EPU48B-41:gapMotorOff", "SR-ID-EPU46-45:gapMotorOff", "SR-ID-EPU48A-41:phaseMotorOff", "SR-ID-EPU48B-41:phaseMotorOff", "SR-ID-EPU46-45:phaseMotorOff"]) -> ("1rst Value (string)"=w311:string[])  [unwired: 8 in, 6 out]
    n130 = To Long Integer(number=w410) -> (32bit integer=w411:i32)
    n131 = To Long Integer(number=w412) -> (32bit integer=w413:i32)
    n132 = To Long Integer(number=w406) -> (32bit integer=w409:i32)
    n133 = To Long Integer(number=w407) -> (32bit integer=w408:i32)
    n134 = Index Array(array=w359, index #1=0 ("index"), index #2=1 ("index"), index #3=2 ("index"), index #4=3 ("index"), index #5=4 ("index"), index #6=5 ("index"), index #7=6 ("index"), index #8=7 ("index"), index #9=8 ("index"), index #10=9 ("index"), index #11=10 ("index"), index #12=11 ("index"), index #13=12 ("index"), index #14=13 ("index"), index #15=14 ("index")) -> (element #1=w256:dbl, element #2=w255:dbl, element #3=w254:dbl, element #4=w253:dbl, element #5=w252:dbl, element #6=w251:dbl, element #7=w250:dbl, element #8=w249:dbl, element #9=w248:dbl, element #10=w247:dbl, element #11=w246:dbl, element #12=w245:dbl, element #13=w244:dbl, element #14=w187:dbl, element #15=w243:dbl)
    n135 = for {
      tunnel: w311 -> [w626] mode=indexing
      tunnel: [w625] -> w310 mode=indexing
      n136 = case shown="\"1\", Default" w626 {
        tunnel: [FALSE TRUE] -> w625
        frame "1", Default {
        }
        frame "0" {
        }
      }
    }
    n137 = Index Array(array=w136, index #1=0 ("index"), index #2=1 ("index"), index #3=2 ("index"), index #4=3 ("index"), index #5=4 ("index"), index #6=5 ("index"), index #7=6 ("index"), index #8=7 ("index"), index #9=8 ("index"), index #10=9 ("index"), index #11=10 ("index"), index #12=11 ("index"), index #13=12 ("index"), index #14=13 ("index"), index #15=14 ("index"), index #16=15 ("index"), index #17=16 ("index"), index #18=17 ("index"), index #19=18 ("index"), index #20=19 ("index"), index #21=20 ("index")) -> (element #1=w133:bool, element #2=w132:bool, element #3=w131:bool, element #4=w120:bool, element #5=w119:bool, element #6=w118:bool, element #7=w113:bool, element #8=w112:bool, element #9=w111:bool, element #10=w102:bool, element #11=w101:bool, element #12=w100:bool, element #13=w95:bool, element #14=w94:bool, element #15=w93:bool, element #16=w92:bool, element #17=w91:bool, element #18=w90:bool, element #19=w89:bool, element #20=w88:bool, element #21=w87:bool)
    n138 = case shown="1" w413 {
      tunnel: [FALSE TRUE] -> w269
      frame 0, Default {
      }
      frame 1 {
      }
    }
    n139 = case shown="1" w408 {
      tunnel: [FALSE TRUE] -> w266
      frame 0, Default {
      }
      frame 1 {
      }
    }
    n140 = case shown="0" w411 {
      tunnel: [TRUE FALSE] -> w268
      frame 0 {
      }
      frame 1, Default {
      }
    }
    n141 = case shown="0" w409 {
      tunnel: [TRUE FALSE] -> w265
      frame 0 {
      }
      frame 1, Default {
      }
    }
    n142 = To Long Integer(number=w474) -> (32bit integer=w477:i32)
    n143 = Negate(x=w187) -> (-x=w186:dbl)
    n144 = case shown="1" w477 {
      tunnel: ["Decay" "Top-Up"] -> w298
      frame 0, Default {
      }
      frame 1 {
      }
    }
    n145 = Index Array(array=w369, index #1=0 ("index"), index #2=1 ("index"), index #3=2 ("index"), index #4=3 ("index"), index #5=4 ("index"), index #6=5 ("index"), index #7=6 ("index")) -> (element #1=w134:bool, element #2=w130:bool, element #3=w114:bool, element #4=w97:bool, element #5=w96:bool, element #6=w78:bool, element #7=w77:bool)
    n146 = case shown="\"MBM\", Default" w387 {
      tunnel: ["MBM" "SBM"] -> w276
      tunnel: w391 -> [w640 _]
      tunnel: [w640 w645] -> w274
      tunnel: w390 -> [_ w645]
      tunnel: w386 -> [_ w644]
      tunnel: w385 -> [w639 _]
      tunnel: [w639 w644] -> w272
      tunnel: w384 -> [_ w643]
      tunnel: w383 -> [w638 _]
      tunnel: [w638 w643] -> w271
      tunnel: w382 -> [_ w642]
      tunnel: w381 -> [w637 _]
      tunnel: [w637 w642] -> w270
      frame "MBM", Default {
      }
      frame "SBM" {
      }
    }
    n147 = Multiply(x=w462, y=w461) -> (x*y=w295:dbl)
    n148 = Divide(x=w457, y=w456) -> (x/y=w293:dbl)
    n149 = Multiply(x=w460, y=w461) -> (x*y=w294:dbl)
    n150 = Divide(x=w455, y=w456) -> (x/y=w292:dbl)
    n151 = Index Array(array=w370, index #1=0 ("index"), index #2=1 ("index"), index #3=2 ("index"), index #4=3 ("index"), index #5=4 ("index"), index #6=5 ("index"), index #7=6 ("index")) -> (element #1=w135:bool, element #2=w129:bool, element #3=w117:bool, element #4=w99:bool, element #5=w98:bool, element #6=w80:bool, element #7=w79:bool)
    n152 = call "FE_PAB_OpenState.vi"("FE"=w135, "XBPMX 2"=w128, "XBPMY 2"=w127, "Hutch"=w134, "PAB"=w133, "MGV"=w132, "FCV"=w131) -> ("XBPMX 2"=w124:string, "XBPMY 2"=w123:string)  [unwired: 7 in]
    n153 = call "FE_PAB_OpenState.vi"("FE"=w129, "XBPMX 2"=w126, "XBPMY 2"=w125, "Hutch"=w130, "PAB"=w120, "MGV"=w119, "FCV"=w118) -> ("XBPMX 2"=w122:string, "XBPMY 2"=w121:string)  [unwired: 7 in]
    n154 = call-poly <userlib>:"CaLabGet.vi"("PV Name"="TI-INJ-PROC:getTrig-SR-KICKER") -> ("1rst Value (string)"=w394:string)  [unwired: 8 in, 6 out]
    n155 = Index Array(array=w310, index #1=0 ("index"), index #2=1 ("index"), index #3=2 ("index"), index #4=3 ("index"), index #5=4 ("index"), index #6=5 ("index"), index #7=6 ("index"), index #8=7 ("index"), index #9=8 ("index"), index #10=9 ("index"), index #11=10 ("index"), index #12=11 ("index"), index #13=12 ("index")) -> (element #1=w228:bool, element #2=w227:bool, element #3=w226:bool, element #4=w225:bool, element #5=w224:bool, element #6=w223:bool, element #7=w222:bool, element #8=w221:bool, element #9=w220:bool, element #10=w219:bool, element #11=w218:bool, element #12=w217:bool, element #13=w216:bool)
    n156 = call-poly <userlib>:"CaLabGet.vi"("PV Names"=w300) -> ("1rst Value (number)"=w302:dbl[])  [unwired: 8 in, 6 out]
    n157 = call-poly <userlib>:"CaLabGet.vi"("PV Names"=w301) -> ("1rst Value (number)"=w304:dbl[])  [unwired: 8 in, 6 out]
    n158 = call "FE_PAB_OpenState.vi"("FE"=w117, "XBPMX 2"=w116, "XBPMY 2"=w115, "Hutch"=w114, "PAB"=w113, "MGV"=w112, "FCV"=w111) -> ("XBPMX 2"=w106:string, "XBPMY 2"=w105:string)  [unwired: 7 in]
    n159 = call-poly <userlib>:"CaLabGet.vi"("PV Names"=string[] ["SR-DI-FOFB-H:getStatus", "SR-DI-FOFB-V:getStatus", "IGPF:TPSX:FBCTRL", "IGPF:TPSY:FBCTRL", "TPS-SR-022:bpm3:ilk:enabled", "SR-DI-ANGLE-ILK:StatusX", "SR-DI-ANGLE-ILK:StatusY"]) -> ("1rst Value (string)"=w202:string[], "1rst Value (number)"=w203:dbl[])  [unwired: 8 in, 5 out]
    n160 = call "FE_PAB_OpenState.vi"("FE"=w99, "XBPMX 2"=w110, "XBPMY 2"=w109, "Hutch"=w97, "PAB"=w102, "MGV"=w101, "FCV"=w100) -> ("XBPMX 2"=w104:string, "XBPMY 2"=w103:string)  [unwired: 7 in]
    n161 = Multiply(x=w302, y=w303) -> (x*y=w176:dbl[])
    n162 = To Byte Integer(number=w203) -> (8bit integer=w199:i8[])
    n163 = Multiply(x=w304, y=w303) -> (x*y=w179:dbl[])
    n164 = for {
      tunnel: w199 -> [w616] mode=indexing
      tunnel: [w615] -> w209 mode=indexing
      n165 = case shown="0, Default" w616 {
        tunnel: [TRUE FALSE] -> w615
        frame 1 {
        }
        frame 0, Default {
        }
      }
    }
    n166 = Array Max & Min(array=w176) -> (max value=w178:dbl, min value=w177:dbl)  [unwired: 2 out]
    n167 = Array Max & Min(array=w179) -> (max value=w181:dbl, min value=w180:dbl)  [unwired: 2 out]
    n168 = call "FE_PAB_OpenState.vi"("FE"=w98, "XBPMX 2"=w108, "XBPMY 2"=w107, "Hutch"=w96, "PAB"=w95, "MGV"=w94, "FCV"=w93) -> ("XBPMX 2"=w86:string, "XBPMY 2"=w85:string)  [unwired: 7 in]
    n169 = Index Array(array=w202, index #1=0 ("index"), index #2=1 ("index")) -> (element #1=w197:string, element #2=w196:string)
    n170 = property on="BPMX Graph" class="XYGraph (strict)"("YScale.Maximum"=w178, "YScale.Minimum"=w177) -> ()  [unwired: 2 in, 2 out]
    n171 = call "FE_PAB_OpenState.vi"("FE"=w80, "XBPMX 2"=w76, "XBPMY 2"=w75, "Hutch"=w78, "PAB"=w92, "MGV"=w91, "FCV"=w90) -> ("XBPMX 2"=w84:string, "XBPMY 2"=w83:string)  [unwired: 7 in]
    n172 = property on="BPMY Graph" class="XYGraph (strict)"("YScale.Maximum"=w181, "YScale.Minimum"=w180) -> ()  [unwired: 2 in, 2 out]
    n173 = call "FE_PAB_OpenState.vi"("FE"=w79, "XBPMX 2"=w74, "XBPMY 2"=w73, "Hutch"=w77, "PAB"=w89, "MGV"=w88, "FCV"=w87) -> ("XBPMX 2"=w82:string, "XBPMY 2"=w81:string)  [unwired: 7 in]
    n174 = Bundle("Array 4"=w305, w176) -> (w215:cluster{"Array 4":i32[], dbl[]})  [unwired: 1 in]
    n175 = Bundle("Array 4"=w305, w179) -> (w214:cluster{"Array 4":i32[], dbl[]})  [unwired: 1 in]
    n176 = Index Array(array=w209, index #1=2 ("index"), index #2=3 ("index"), index #3=4 ("index"), index #4=5 ("index"), index #5=6 ("index")) -> (element #1=w195:bool, element #2=w194:bool, element #3=w193:bool)  [unwired: 2 out]
    n177 = Equal?(x="1" ("1rst Value (string)"), y=w394) -> (x = y?=w392:bool)
    "x = y?" <- w392
    n178 = case shown="False" w392 {
      tunnel: w459 -> [_ w650]
      tunnel: w458 -> [_ w649]
      tunnel: [w648 w650] -> w185
      tunnel: [w647 w649] -> w184
      tunnel: w183 -> [w648 _]
      tunnel: w182 -> [w647 _]
      frame False {
      }
      frame True {
        n179 = local read "NOW date"() -> (→"date kickeron":string)
        n180 = local read "NOW time"() -> (→"time kickeron":string)
      }
    }
    n181 = Wait Until Next ms Multiple(millisecond multiple=u32 1000) -> ()  [unwired: 1 out]
    n182 = local read "date kickeron"() -> (w191:string)
    n183 = local read "time kickeron"() -> (w190:string)
    n184 = Get Date/Time In Seconds() -> (seconds since 1Jan1904=w307:timestamp)
    n185 = call-poly <userlib>:"CaLabGet.vi"("PV Names"=w72) -> ("1rst Value (string)"=w61:string[])  [unwired: 8 in, 6 out]
    n186 = Format Date/Time String(time format string (%c)="%Y/%m/%d", seconds (now)=w307) -> (date/time string=→"NOW date":string)  [unwired: 1 in]
    n187 = Format Date/Time String(time format string (%c)="%Y/%m/%d", seconds (now)=w307) -> (date/time string=w213:string)  [unwired: 1 in]
    n188 = Format Date/Time String(time format string (%c)="%H:%M:%S", seconds (now)=w307) -> (date/time string=w212:string)  [unwired: 1 in]
    "NOW time" <- w212
    n189 = Index Array(array=w61, index #1=0 ("index"), index #2=1 ("index"), index #3=2 ("index"), index #4=3 ("index"), index #5=4 ("index"), index #6=5 ("index"), index #7=6 ("index"), index #8=7 ("index"), index #9=8 ("index"), index #10=9 ("index")) -> (element #1=w60:string, element #2=w59:string, element #3=w58:string, element #4=w57:string, element #5=w56:string, element #6=w55:string, element #7=w54:string, element #8=w53:string, element #9=w52:string, element #10=w51:string)
    n190 = Bundle By Name(cluster=T4 {"SR Fill Pattern"=array[864 elements], "Beam Current(mA"=301.91562200000004, "Beam Lifetime(min)"=669.1065769463743, "Beamsize X(um)"=55.54579477590784, "Beamsize Y(um)"=33.648665625479325, "Tune X(from BPM)"=0.1399, "Tune Y(from BPM)"=0.14, "Mode"="Top-Up", "NuX(from BBF) "=0.16718639681347974, "NuY(from BBF)"=0.25219386232318686, "IU22-23gap(R)"=11.0, "IU22-05gap(R)"=7.558, "IU22-05M"=TRUE, "IU22A-09gap(R)"=8.075, "IU22A-09M"=TRUE, "IU22B-09gap(R)"=40.001, "IU22B-09M"=FALSE, "IUT22-21gap(R)"=7.0, "IUT22-21M"=TRUE, "IU22-23M"=TRUE, "IU22A-25gap(R)"=8.18, "IU22A-25M"=TRUE, "IU22B-25gap(R)"=40.0, "IU22B-25M"=FALSE, "EPU48A-41gap(R)"=64.99985000000001, "EPU48A-41gM"=TRUE, "EPU48B-41gap(R)"=65.00399999999999, "EPU48B-41gM"=FALSE, "EPU46-45gap(R)"=45.00005, "EPU46-45gM"=TRUE, "EPU48A-41phase(R)"=0.0001, "EPU48B-41phase(R)"=0.00055, "EPU46-45phase(R)"=0.0, "Grid volt.(V)(S)"=33.0, "Gun mode"="MBM", "Mod.3 HV(kV)(S)"=35.800000000000026, "SR"="SR_DMB_2016_1102_1124LOCO.data", "BR"="Booster_JT_2016_1005_1200.data", "Linac"="Linac2016_1005_0935.data", "LTB"="LTB_JT_2016_1005_1200.data", "BTS"="BTS_2016_1116_1020.data", "RF2 remote"=TRUE, "RF2 OP mode"=TRUE, "RF2 phase.(S)"=-56.70000000000001, "RF Freq.(s)"=499654660.62238467, "RF2 gap volt.(S)"=1400.0, "RF3 remote"=TRUE, "RF3 OP mode"=TRUE, "RF3 phase.(S)"=160.0, "RF3 gap volt.(S)"=1400.0, "BBF V"=TRUE, "BBF H"=TRUE, "BR ext. kicker1(kV)"=18.266, "BR ext. kicker2(kV)"=18.26600000000001, "BR ext. sep.1(V)"=318.8444, "BR ext. sep.2(V)"=444.5, "BR inj. sep.(V)"=105.2, "BR inj. kicker(kV)"=16.40000000000001, "SR kicker4(kV)"=8.27, "SR kicker3(kV)"=8.315, "SR kicker2(kV)"=8.325, "SR kicker1(kV)"=8.4, "SR inj. sep.2(V)"=417.0, "SR inj. sep.1(V)"=419.3416, "Bucket Start"=100.0, "Bucket Last"=630.0, "Bucket Step"=10.0, "Orbit ILK(P)"=TRUE, "IU22-05 Hutch Enable"=TRUE, "IU22A-09M Hutch Enable"=TRUE, "IUT22-21M Hutch Enable"=TRUE, "IU22-23M Hutch Enable"=FALSE, "IU22A-25M Hutch Enable"=TRUE, "EPU48A-41M Hutch Enable"=FALSE, "EPU46-45M Hutch Enable"=TRUE, "EPU46-45 FE Enable"=TRUE, "EPU48A-41 FE Enable"=FALSE, "IU22A-25 FE Enable"=TRUE, "IU22-23 FE Enable"=FALSE, "IUT22-21 FE Enable"=TRUE, "IU22A-09 FE Enable"=TRUE, "IU22-05 FE Enable"=TRUE, "EPU48A-41pM"=TRUE, "EPU48B-41pM"=FALSE, "EPU46-45pM"=FALSE, "Gun volt.(V)(S)"=23.5, "Width count"=30.0, "2ns step"=0.0, "10ps delay"=100.0, "phase shifter"=130.00060000000002, "Taper"=-1.0899999999999999, "05XBPMX 1"=115.877, "09XBPMX 1"=471.421, "21XBPMX 1"=612.331, "23XBPMX 1"=-46.736000000000004, "25XBPMX 1"=462.29900000000004, "41XBPMX 1"=364.139, "45XBPMX 1"=-164.196, "05XBPMY 1"=-62.875, "09XBPMY 1"=-23.034, "21XBPMY 1"=-27.449, "23XBPMY 1"=-89.72200000000001, "25XBPMY 1"=459.291, "41XBPMY 1"=-111.624, "45XBPMY 1"=-57.689, "FOFB H"="On", "FOFB V"="On", "time string"="21:36:25", "date"="2016/11/21", "date (last kicker ON)"="wait to fire", "time string (last kicker ON)"="", "BPMX Graph"={[1, 2, 3, 4, 5, 6, 7, 8, 9, 10, 11, 12, 13, 14, 15, 16, 17, 18, 19, 20, 21, 22, 23, 24, 25, 26, 27, 28, 29, 30, 31, 32, 33, 34, 35, 36, 37, 38, 39, 40, 41, 42, 43, 44, 45, 46, 47, 48, 49, 50, 51, 52, 53, 54, 55, 56, 57, 58, 59, 60, 61, 62, 63, 64, 65, 66, 67, 68, 69, 70, 71, 72, 73, 74, 75, 76, 77, 78, 79, 80, 81, 82, 83, 84, 85, 86, 87, 88, 89, 90, 91, 92, 93, 94, 95, 96, 97, 98, 99, 100, 101, 102, 103, 104, 105, 106, 107, 108, 109, 110, 111, 112, 113, 114, 115, 116, 117, 118, 119, 120, 121, 122, 123, 124, 125, 126, 127, 128, 129, 130, 131, 132, 133, 134, 135, 136, 137, 138, 139, 140, 141, 142, 143, 144, 145, 146, 147, 148, 149, 150, 151, 152, 153, 154, 155, 156, 157, 158, 159, 160, 161, 162, 163, 164, 165, 166, 167, 168, 169, 170, 171, 172, 173, 174], "1rst Value (number)"=[-31.198, -3.303, -73.172, -2.032, 86.386, -75.851, 71.519, -46.03, 6.824, -37.804, 68.275, -4.672, -223.404, -16.867, -6.964, -259.448, -62.697, 1.8880000000000001, 75.267, -92.668, 86.714, -30.843, 12.767, -107.398, -44.436, 161.126, 208.922, 211.488, -27.247, 79.489, 826.962, 470.705, -115.522, -41.497, 159.486, -54.261, -0.64, 42.641, -2.466, -143.394, -24.785, 138.912, -65.805, 42.325, 32.891, -7.298, -96.724, -31.725, 98.531, -80.64, 64.163, 94.83, -44.03, -163.192, 50.589, 46.669000000000004, -87.508, 78.479, 31.618000000000002, -17.077, -125.32600000000001, -3.845, 98.34100000000001, -39.679, 50.247, -58.208, 40.297000000000004, -69.857, 42.548, -19.403, -211.0, -9.082, -322.597, -233.847, -140.75, 97.087, -15.869, -29.053, 59.46, -115.316, 70.896, -60.685, 33.715, 12.09, -520.422, -138.423, -302.753, 79.862, 120.014, 122.671, -55.812, 27.084, 39.115, -138.936, 156.631, 53.777, -72.647, -52.588, 16.002, 45.197, -117.489, 121.709, 27.952, -31.609, -113.58500000000001, 45.019, 55.136, -130.553, 138.93200000000002, 35.998, -30.631, -96.529, -7.589, 100.395, -93.919, 40.569, 79.538, -68.044, -134.578, 2.52, 84.539, -59.166000000000004, 42.576, 34.657000000000004, -15.805, -52.158, 18.484, 4.346, -157.404, 182.672, 202.518, -164.868, -53.871, 8.066, -9.738, -55.594, 92.623, -13.785, 11.587, -60.627, -47.704, 65.516, 57.924, 148.347, -201.348, -302.753, 189.117, 72.681, -134.928, 39.791000000000004, 45.938, -49.072, 54.473, 28.991, -20.657, -80.283, -20.264, 106.907, -121.271, 150.281, -2.243, -11.844, -122.82300000000001, 0.973, 114.186, -107.94, 95.485, 40.314, -36.956, -134.537, 16.196, 91.88, -35.505, -0.018000000000000002]}, "BPMY Graph"={[1, 2, 3, 4, 5, 6, 7, 8, 9, 10, 11, 12, 13, 14, 15, 16, 17, 18, 19, 20, 21, 22, 23, 24, 25, 26, 27, 28, 29, 30, 31, 32, 33, 34, 35, 36, 37, 38, 39, 40, 41, 42, 43, 44, 45, 46, 47, 48, 49, 50, 51, 52, 53, 54, 55, 56, 57, 58, 59, 60, 61, 62, 63, 64, 65, 66, 67, 68, 69, 70, 71, 72, 73, 74, 75, 76, 77, 78, 79, 80, 81, 82, 83, 84, 85, 86, 87, 88, 89, 90, 91, 92, 93, 94, 95, 96, 97, 98, 99, 100, 101, 102, 103, 104, 105, 106, 107, 108, 109, 110, 111, 112, 113, 114, 115, 116, 117, 118, 119, 120, 121, 122, 123, 124, 125, 126, 127, 128, 129, 130, 131, 132, 133, 134, 135, 136, 137, 138, 139, 140, 141, 142, 143, 144, 145, 146, 147, 148, 149, 150, 151, 152, 153, 154, 155, 156, 157, 158, 159, 160, 161, 162, 163, 164, 165, 166, 167, 168, 169, 170, 171, 172, 173, 174], "1rst Value (number)"=[-99.743, 2.851, -30.024, 83.777, -46.733000000000004, -39.889, 2.349, -4.944, 17.022000000000002, 9.824, 11.632, 41.188, -13.992, 13.911, -6.211, 53.857, -48.993, -32.789, -6.3740000000000006, -62.867000000000004, -8.332, 72.09400000000001, -75.398, 53.283, 63.008, -2.23, 43.024, 32.073, -246.641, -93.162, 456.41700000000003, 88.299, 58.803000000000004, 1.7590000000000001, 35.664, 6.575, 18.59, -30.439, 11.254, -28.256, -62.707, -4.503, 1.31, -21.571, 34.77, -8.876, 31.237000000000002, 25.402, 2.726, 20.655, -7.845, -1.443, -31.935000000000002, -16.981, 13.022, 17.515, -82.867, 61.285000000000004, -57.573, 110.363, -27.753, 28.322, -9.241, 53.929, -25.816, 24.231, -57.876, -11.578, 32.087, -70.84, 64.43, 9.409, -157.639, -57.0, 39.267, 30.23, 18.993000000000002, -33.97, 26.195, -10.585, -17.617, -18.667, 31.615000000000002, -25.437, 29.564, 13.537, 6.728, 163.38400000000001, 106.51, -70.056, 12.874, -4.125, -10.855, -21.856, 1.947, 8.096, 11.402000000000001, 5.761, 41.929, -8.752, 18.634, 7.553, -40.034, 39.183, -25.067, -32.557, 5.393, -17.564, -1.614, 20.498, -14.818, 10.313, 35.254, -35.886, 58.359, -36.56, -20.354, 7.593, -21.256, -8.001, -16.79, 10.18, -16.327, 20.416, -10.539, 19.944, -6.801, 13.068, -13.644, 3.468, -0.983, -17.6, 6.785, -26.101, -11.52, 61.191, -32.777, 13.536, 4.026, -14.682, 52.057, -53.883, 27.118000000000002, 31.672, 79.62, 17.715, 15.693, 113.157, -57.095, 14.214, -4.787, -11.148, -3.157, -6.251, -0.764, 3.563, 7.3500000000000005, 10.779, 21.129, 11.36, 7.771, -14.787, -13.278, 0.279, -13.516, -62.422000000000004, -13.389000000000001, 80.56400000000001, -108.465, 69.885, 30.116, 21.421, 32.779, -10.527000000000001]}, "Radio Buttons 2"=enum."absolute", "09XBPMX 2"="", "09XBPMY 2"="", "05XBPMY 2"="", "05XBPMX 2"="", "21XBPMY 2"="", "21XBPMX 2"="", "23XBPMY 2"="", "23XBPMX 2"="", "25XBPMY 2"="", "25XBPMX 2"="", "41XBPMY 2"="", "41XBPMX 2"="", "45XBPMX 2"="", "45XBPMY 2"="", "05 mode"="", "09A mode"="", "09B mode"="", "21 mode"="", "23 mode"="", "25A mode"="", "25B mode"="", "41A mode"="", "41B mode"="", "46 mode"="", "BeamCurrent History"={"BPM NO.  1_172"=[3587880327.0, 3587880337.0, 3587880347.0, 3587880357.0, 3587880367.0, 3587880377.0, 3587880388.0, 3587880398.0, 3587880408.0, 3587880417.0, 3587880427.0, 3587880437.0, 3587880447.0, 3587880457.0, 3587880467.0, 3587880477.0, 3587880487.0, 3587880497.0, 3587880507.0, 3587880517.0, 3587880527.0, 3587880537.0, 3587880547.0, 3587880557.0, 3587880567.0, 3587880577.0, 3587880587.0, 3587880597.0, 3587880607.0, 3587880617.0, 3587880627.0, 3587880637.0, 3587880647.0, 3587880657.0, 3587880667.0, 3587880677.0, 3587880687.0, 3587880697.0, 3587880707.0, 3587880717.0, 3587880727.0, 3587880737.0, 3587880747.0, 3587880757.0, 3587880767.0, 3587880777.0, 3587880787.0, 3587880797.0, 3587880807.0, 3587880817.0, 3587880827.0, 3587880837.0, 3587880847.0, 3587880857.0, 3587880867.0, 3587880877.0, 3587880887.0, 3587880897.0, 3587880907.0, 3587880917.0], [279.8706, 279.6878, 279.5138, 279.3326, 279.1537, 278.9744, 280.1668, 279.9874, 279.8097, 279.6281, 279.4484, 279.2734, 279.0933, 279.9395, 280.0027, 279.8235, 279.642, 279.4661, 279.2873, 279.1089, 279.6484, 280.0044, 279.8243, 279.6482, 279.4694, 279.2899, 279.1109, 279.5519, 279.9906, 279.8127, 279.6339, 279.4608, 279.2828, 279.104, 279.6982, 279.9463, 279.7671, 279.5915, 279.4126, 279.2368, 279.0606, 280.1311, 279.9543, 279.7767, 279.6011, 279.4247, 279.2452, 279.0726, 280.2098, 280.0333, 279.8566, 279.6814, 279.5039, 279.3286, 279.1559, 278.9767, 280.1638, 279.9891, 279.8148, 279.6383]}, "SR Beam Current in Last           Hrs"=12.0} ("Cluster"), "Tune X(from BPM)"=w185, "Tune Y(from BPM)"=w184, "date (last kicker ON)"=w191, "time string (last kicker ON)"=w190, "date"=w213, "time string"=w212, "Mode"=w298, "Beam Current(mA"=w297, "Beam Lifetime(min)"=w296, "Beamsize X(um)"=w295, "Beamsize Y(um)"=w294, "NuX(from BBF)"=w293, "NuY(from BBF)"=w292, "Bucket Start"=w291, "Bucket Last"=w290, "Bucket Step"=w289, "BR inj. sep.(V)"=w288, "BR inj. kicker(kV)"=w287, "BR ext. kicker1(kV)"=w286, "BR ext. kicker2(kV)"=w285, "BR ext. sep.1(V)"=w284, "BR ext. sep.2(V)"=w283, "SR inj. sep.1(V)"=w282, "SR inj. sep.2(V)"=w281, "SR kicker1(kV)"=w280, "SR kicker2(kV)"=w279, "SR kicker3(kV)"=w278, "SR kicker4(kV)"=w277, "Gun mode"=w276, "Grid volt.(V)(S)"=w275, "Gun volt.(V)(S)"=w274, "Mod.3 HV(kV)(S)"=w273, "Width count"=w272, "2ns step"=w271, "10ps delay"=w270, "RF2 remote"=w269, "RF2 OP mode"=w268, "RF2 phase.(S)"=w189, "RF Freq.(s)"=w267, "RF2 gap volt.(S)"=w188, "RF3 remote"=w266, "RF3 OP mode"=w265, "RF3 phase.(S)"=w264, "RF3 gap volt.(S)"=w263, "BR"=w262, "BTS"=w261, "Linac"=w259, "LTB"=w258, "SR"=w260, "SR Fill Pattern"=w257, "IU22-05 Hutch Enable"=w134, "IU22A-09M Hutch Enable"=w130, "IUT22-21M Hutch Enable"=w114, "IU22-23M Hutch Enable"=w97, "IU22A-25M Hutch Enable"=w96, "EPU48A-41M Hutch Enable"=w78, "EPU46-45M Hutch Enable"=w77, "EPU46-45 FE Enable"=w79, "EPU48A-41 FE Enable"=w80, "IU22A-25 FE Enable"=w98, "IU22-23 FE Enable"=w99, "IUT22-21 FE Enable"=w117, "IU22A-09 FE Enable"=w129, "IU22-05 FE Enable"=w135, "IU22-05gap(R)"=w256, "IU22A-09gap(R)"=w255, "IU22B-09gap(R)"=w254, "IUT22-21gap(R)"=w253, "IU22-23gap(R)"=w252, "IU22A-25gap(R)"=w251, "IU22B-25gap(R)"=w250, "EPU48A-41gap(R)"=w249, "EPU48A-41phase(R)"=w248, "EPU48B-41gap(R)"=w247, "EPU48B-41phase(R)"=w246, "EPU46-45gap(R)"=w245, "EPU46-45phase(R)"=w244, "Taper"=w186, "phase shifter"=w243, "05XBPMX 1"=w242, "09XBPMX 1"=w241, "21XBPMX 1"=w240, "23XBPMX 1"=w239, "25XBPMX 1"=w238, "41XBPMX 1"=w237, "45XBPMX 1"=w236, "05XBPMY 1"=w235, "09XBPMY 1"=w234, "21XBPMY 1"=w233, "23XBPMY 1"=w232, "25XBPMY 1"=w231, "41XBPMY 1"=w230, "45XBPMY 1"=w229, "IU22-05M"=w228, "IU22A-09M"=w227, "IU22B-09M"=w226, "IUT22-21M"=w225, "IU22-23M"=w224, "IU22A-25M"=w223, "IU22B-25M"=w222, "EPU48A-41gM"=w221, "EPU48B-41gM"=w220, "EPU46-45gM"=w219, "EPU48A-41pM"=w218, "EPU48B-41pM"=w217, "EPU46-45pM"=w216, "BPMX Graph"=w215, "BPMY Graph"=w214, "Radio Buttons 2"=enum32{"absolute", "different with"}."absolute", "FOFB H"=w197, "FOFB V"=w196, "BBF H"=w195, "BBF V"=w194, "Orbit ILK(P)"=w193, "05XBPMX 2"=w124, "05XBPMY 2"=w123, "09XBPMX 2"=w122, "09XBPMY 2"=w121, "21XBPMX 2"=w106, "21XBPMY 2"=w105, "23XBPMX 2"=w104, "23XBPMY 2"=w103, "25XBPMX 2"=w86, "25XBPMY 2"=w85, "41XBPMX 2"=w84, "41XBPMY 2"=w83, "45XBPMX 2"=w82, "45XBPMY 2"=w81, "05 mode"=w60, "09A mode"=w59, "09B mode"=w58, "21 mode"=w57, "23 mode"=w56, "25A mode"=w55, "25B mode"=w54, "41A mode"=w53, "41B mode"=w52, "46 mode"=w51, "BeamCurrent History"=w45) -> (→"Cluster":T4)
    n191 = case shown="True" TRUE {
      tunnel: w46 -> [_ w481]
      frame False {
      }
      frame True {
        n192 = Quit LabVIEW(quit? (T)=w481) -> ()
      }
    }
  }
  n193 = local write "stop"(FALSE ("stop")) -> ()
